vi "NEW数据采集传输系统.vi"() -> ()   [LabVIEW 2016, in "数据传输系统.lvlib"]
uses:
  <vilib>/Averna/Notify Icon/NotifyIcon.llb/BalloonIcon.ctl
  <vilib>/Utility/miscctls.llb/LVPointTypeDef.ctl
  <vilib>/Utility/config.llb/Read Key (String).vi
  <vilib>/Averna/Notify Icon/NotifyIcon.llb/GetSelectedItemEvent.vi
  <vilib>/Averna/Notify Icon/NotifyIcon.llb/SetVisible.vi
  <vilib>/Averna/Notify Icon/NotifyIcon.llb/SetMenuDefaultItem.vi
  <vilib>/Averna/Notify Icon/NotifyIcon.llb/SetTipText.vi
  <vilib>/Utility/config.llb/NI_LVConfig.lvlib
  data/FreeMem.dll
  <vilib>/Averna/Notify Icon/NotifyIcon.llb/NotifyIcon.lvclass
  <vilib>/ptbypt/NI_PtbyPt.lvlib
panel:
  in  "updateconfiguration":T1={"主机"="27.154.58.30", "用户"="update", "密码"="std23506", "远程路径"="数据传输系统\\平台数据传输系统.exe", "下载文件名"="平台数据传输系统.exe", "软件版本"=""}
  out "标题显示":string
  in  "更新":bool
  out "错误输出":errorcluster
  in  "停止输入":bool caption="停止 2"
  in  "系统编码选择框":string(combo)="地表水质量监测"
  in  "数据发送通道":enum16{"TCP", "VISA"}(ring)
  in  "baud rate":u32=9600 caption="波特率"
  in  "VISA resource name":refnum<visa-resource-name> caption="VISA资源名称"
  in  "实时数据发送时间间隔/min":i32=1
  in  "数据组合发送":bool
  in  "日志、参数发送":bool
  in  "2011发送":bool
  in  "判断数据反馈":bool
  in  "数据发送协议":enum16{"2005-212协议", "2017-212协议"}(ring)=enum."2017-212协议"
  in  "重发时间":T2(ring)
  in  "重发日期":T3(ring)
  in  "开机启动":bool
  in  "确定更改起始时间":bool
  in  "更改起始时间":bool
  in  "数据发送起始时间":timestamp format="%<%.3X\n%Y/%m/%d>T"
  in  "每周自动重发":bool=TRUE
  in  "确定":bool
  in  "返回":bool
  in  "PW":string
  in  "MN":string
  in  "PORT":string
  in  "IP":string
  in  "站点设备":string
  in  "站点名称":string
  out "设置超时时间/min":i32=1
  out "状态信息":T4={"1st Error to Convert "=63, "步骤 "=enum."发送数据", "元素"="实时数据", "TCP服务端掉线计数"=0, "TCP掉线时间节点"="2019/05/08 15:24:17"} {"1st Error to Convert" items=["无错误", "参数错误", "内存已满", "超出区域", "文件结束", "文件已打开", "一般文件IO错误", "未找到文件", "文件权限错误", "磁盘已满", "路径副本", "打开过多文件", "未启用", "未找到资源文件", "无法添加资源", "未找到资源", "未找到图像", "图像内存错误", "画笔不存在", "配置错误类型", "配置未找到解析段", "配置解析错误", "配置内存错误", "错误外部代码格式", "错误外部代码偏移量", "外部代码不存在", "空窗口", "销毁窗口错误", "空菜单", "打印已中止", "错误打印记录", "打印驱动程序错误", "打印时窗口错误", "打印时内存错误", "打印对话框错误", "一般打印错误", "无效设备引用句柄", "设备未找到", "设备参数错误", "设备单位错误", "无法打开设备", "设备调用已中止", "一般错误", "用户已取消", "对象ID过低", "对象ID过高", "对象不在堆中", "未知的堆", "错误DefProc ID", "DefProc不在表格中", "范围外信息", "空方法", "未知信息", "不支持管理器调用", "错误地址", "连接过程中", "连接超时", "连接过程中", "不支持网络属性", "网络错误", "正在使用的地址", "系统缺少内存", "连接已中止", "连接已拒绝", "连接未建立", "连接已建立", "连接已关闭", "初始化错误（交互应用程序管理器）", "错误事件发生", "等待无约束事件发生处理程序", "事件发生队列溢出", "错误路径", "未发出信号量", "未识别类型（交互应用程序管理器）"]}
  out "数据接收超时指示灯":bool
  out "空闲时间/s":string
  out "系统时间":string
  out "实时小时数据上传":bool
  out "系统状态改变":bool
  out "软件版本":string
  out "掉线指示":bool
  out "核查数据上传":bool
  out "配置信息":T5
  in  "参数配置":bool
  out "反控数据发送":bool
  out "读取报文显示":string
  out "发送报文显示":string
  out "心跳包":bool
  out "通信状态":bool
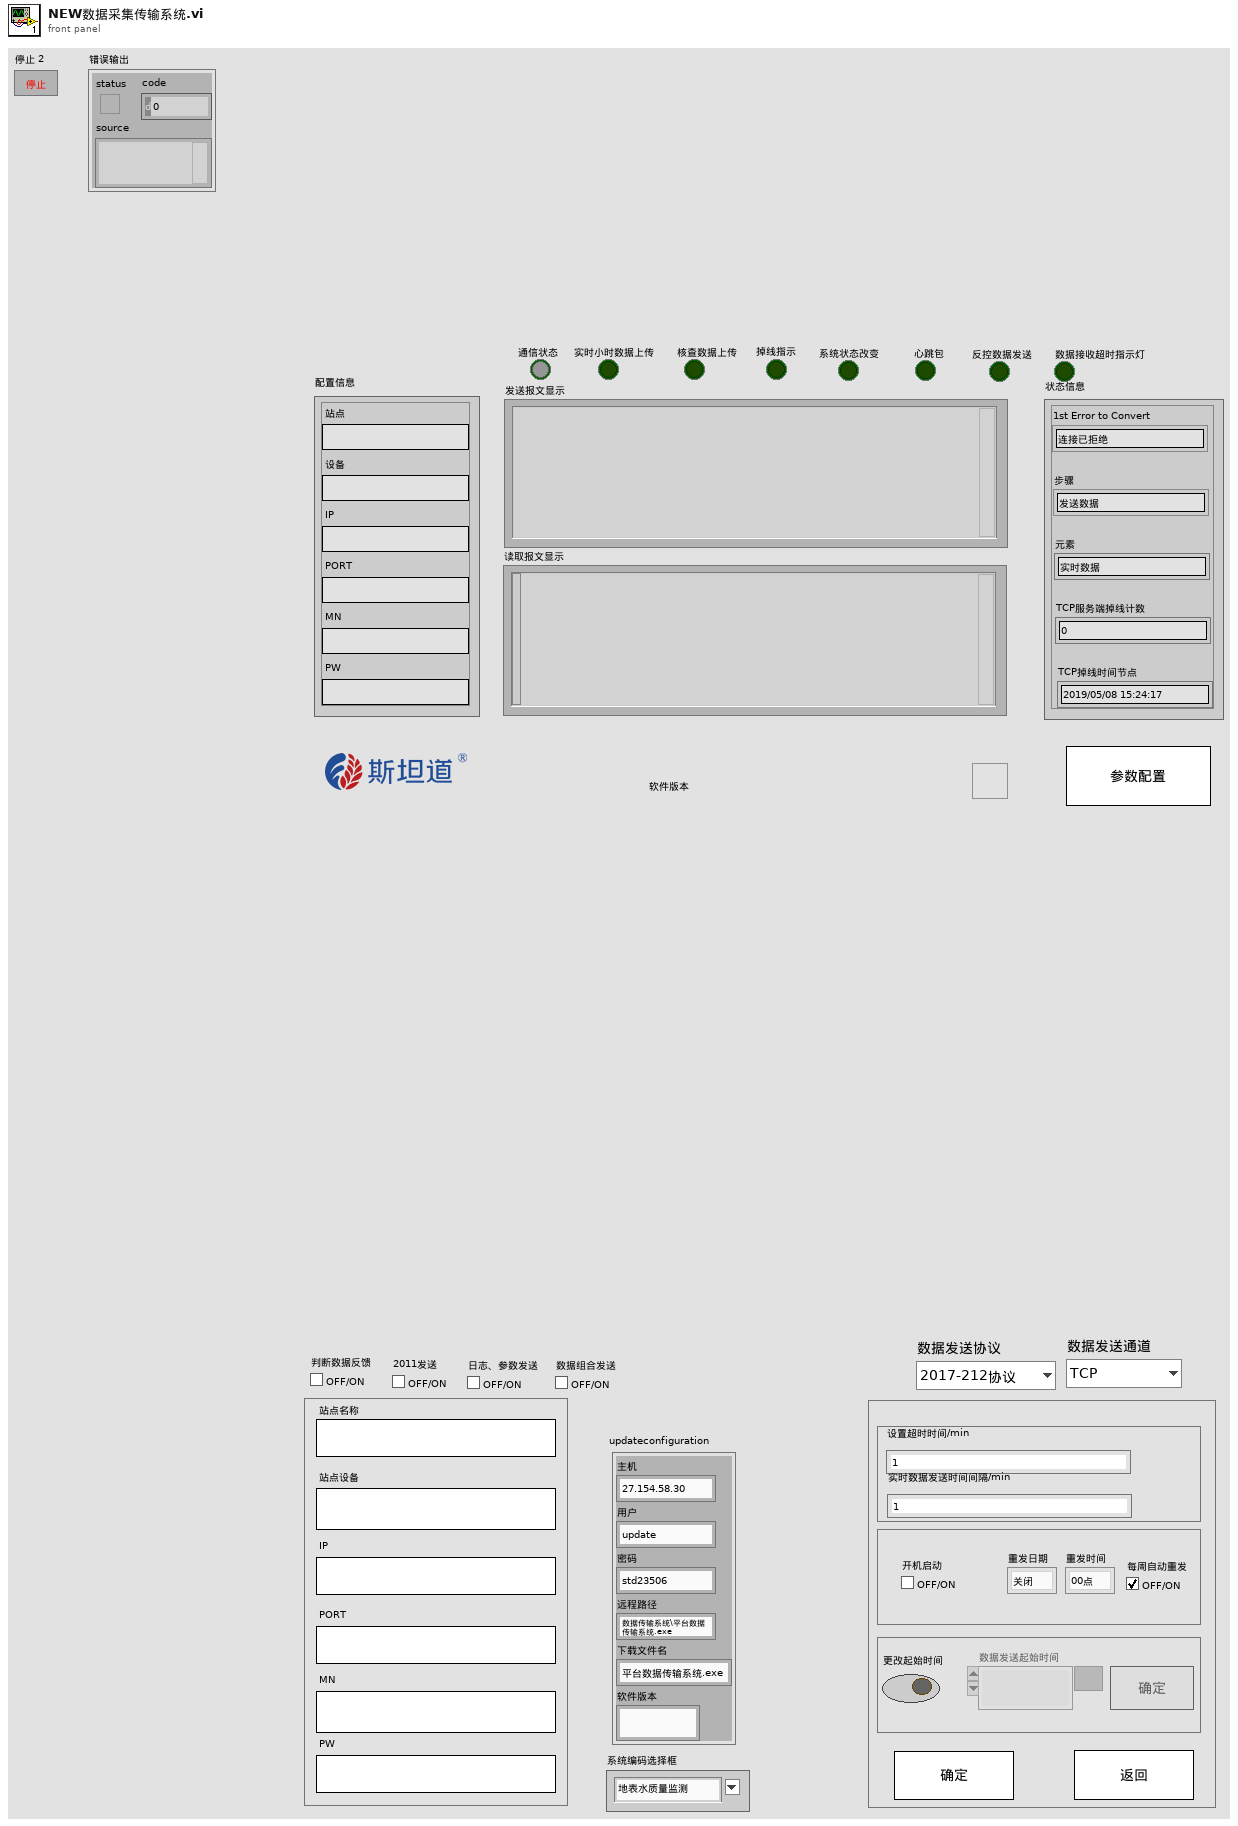
[diagram p1: front panel]
types:
  T1 = cluster{"主机":string, "用户":string, "密码":string, "远程路径":string, "下载文件名":string, "软件版本":string}
  T2 = enum16{"00点", "01点", "02点", "03点", "04点", "05点", "06点", "07点", "08点", "09点", "10点", "11点", "12点", "13点", "14点", "15点", "16点", "17点", "18点", "19点", "20点", "21点", "22点", "23点"}
  T3 = enum16{"关闭", "星期日", "星期一", "星期二", "星期三", "星期四", "星期五", "星期六"}
  T4 = cluster{"1st Error to Convert ":i32, "步骤 ":enum16{"打开连接", "发送数据", "读取数据", "数据处理", "关闭连接"}, "元素":string, "TCP服务端掉线计数":i32, "TCP掉线时间节点":string}
  T5 = cluster{"站点":string, "设备":string, "IP":string, "PORT":string, "MN":string, "PW":string}
  T6 = typedef "LVDateTimeRec.ctl" = cluster{"秒数的小数部分":dbl, "秒":i32, "分":i32, "时":i32, "日":i32, "月":i32, "年":i32, "天数（周）":i32, "天数（年）":i32, "DST":i32}
  T7 = enum32{"invalid app kind", "Development System", "Run Time System", "Student Edition", "Embedded LabVIEW", "Evaluation", "Custom"}
  T8 = typedef "LVPointTypeDef.ctl" = cluster{"Horizontal":i16, "Vertical":i16}
  T9 = cluster{"CODMn":bool, "CODCr":bool, "DO":bool, "铜":bool, "PH":bool, "氨氮":bool, "比电导率":bool, "水温":bool, "COD":bool, "浊度":bool, "总氮":bool, "总磷":bool, "叶绿素a":bool, "藻密度":bool, "水位":bool, "流速":bool, "瞬时流量":bool, "累积流量":bool, "亚硝酸盐":bool, "硫化物":bool, "ORP":bool, "铅":bool, "镉":bool, "锌":bool, "镍":bool, "锰":bool, "汞":bool}
  T10 = typedef "NI_LVConfig.lvlib/Config Data RefNum.ctl" = refnum<k1>
  T11 = typedef "imagedata.ctl" = cluster{"image type":i32, "image depth":i32, "image":u8[], "mask":u8[], "colors":u32[], "Rectangle":cluster{"left":i16, "top":i16, "right":i16, "bottom":i16}}
  T12 = cluster{"[0]":string, "[1]":string, "[2]":string, "[3]":string, "[4]":string, "[5]":string, "[6]":string, "[7]":string, "[8]":string, "[9]":string, "[10]":string, "[11]":string, "[12]":string, "[13]":string, "[14]":string, "[15]":string, "[16]":string, "[17]":string, "[18]":string, "[19]":string, "[20]":string, "[21]":string, "[22]":string, "[23]":string, "[24]":string, "[25]":string, "[26]":string}
  T13 = enum8{"Enabled", "Disabled", "Disabled and Grayed Out"}
  T14 = cluster{"[0]":string, "[1]":string, "[2]":string, "[3]":string, "[4]":string, "[5]":string, "[6]":string, "[7]":string}
  T15 = cluster{"[0]":string, "[1]":string, "[2]":string, "[3]":string, "[4]":string, "[5]":string, "[6]":string, "[7]":string, "[8]":string, "[9]":string, "[10]":string, "[11]":string, "[12]":string, "[13]":string, "[14]":string}
  T16 = enum32{"Invalid", "Standard", "Closed", "Hidden", "Minimized", "Maximized"}
  T17 = typedef "NotifyIcon.lvlib/NotifyIcon.lvclass/BalloonIcon.ctl" = enum32{"None", "Information", "Warning", "Error"}
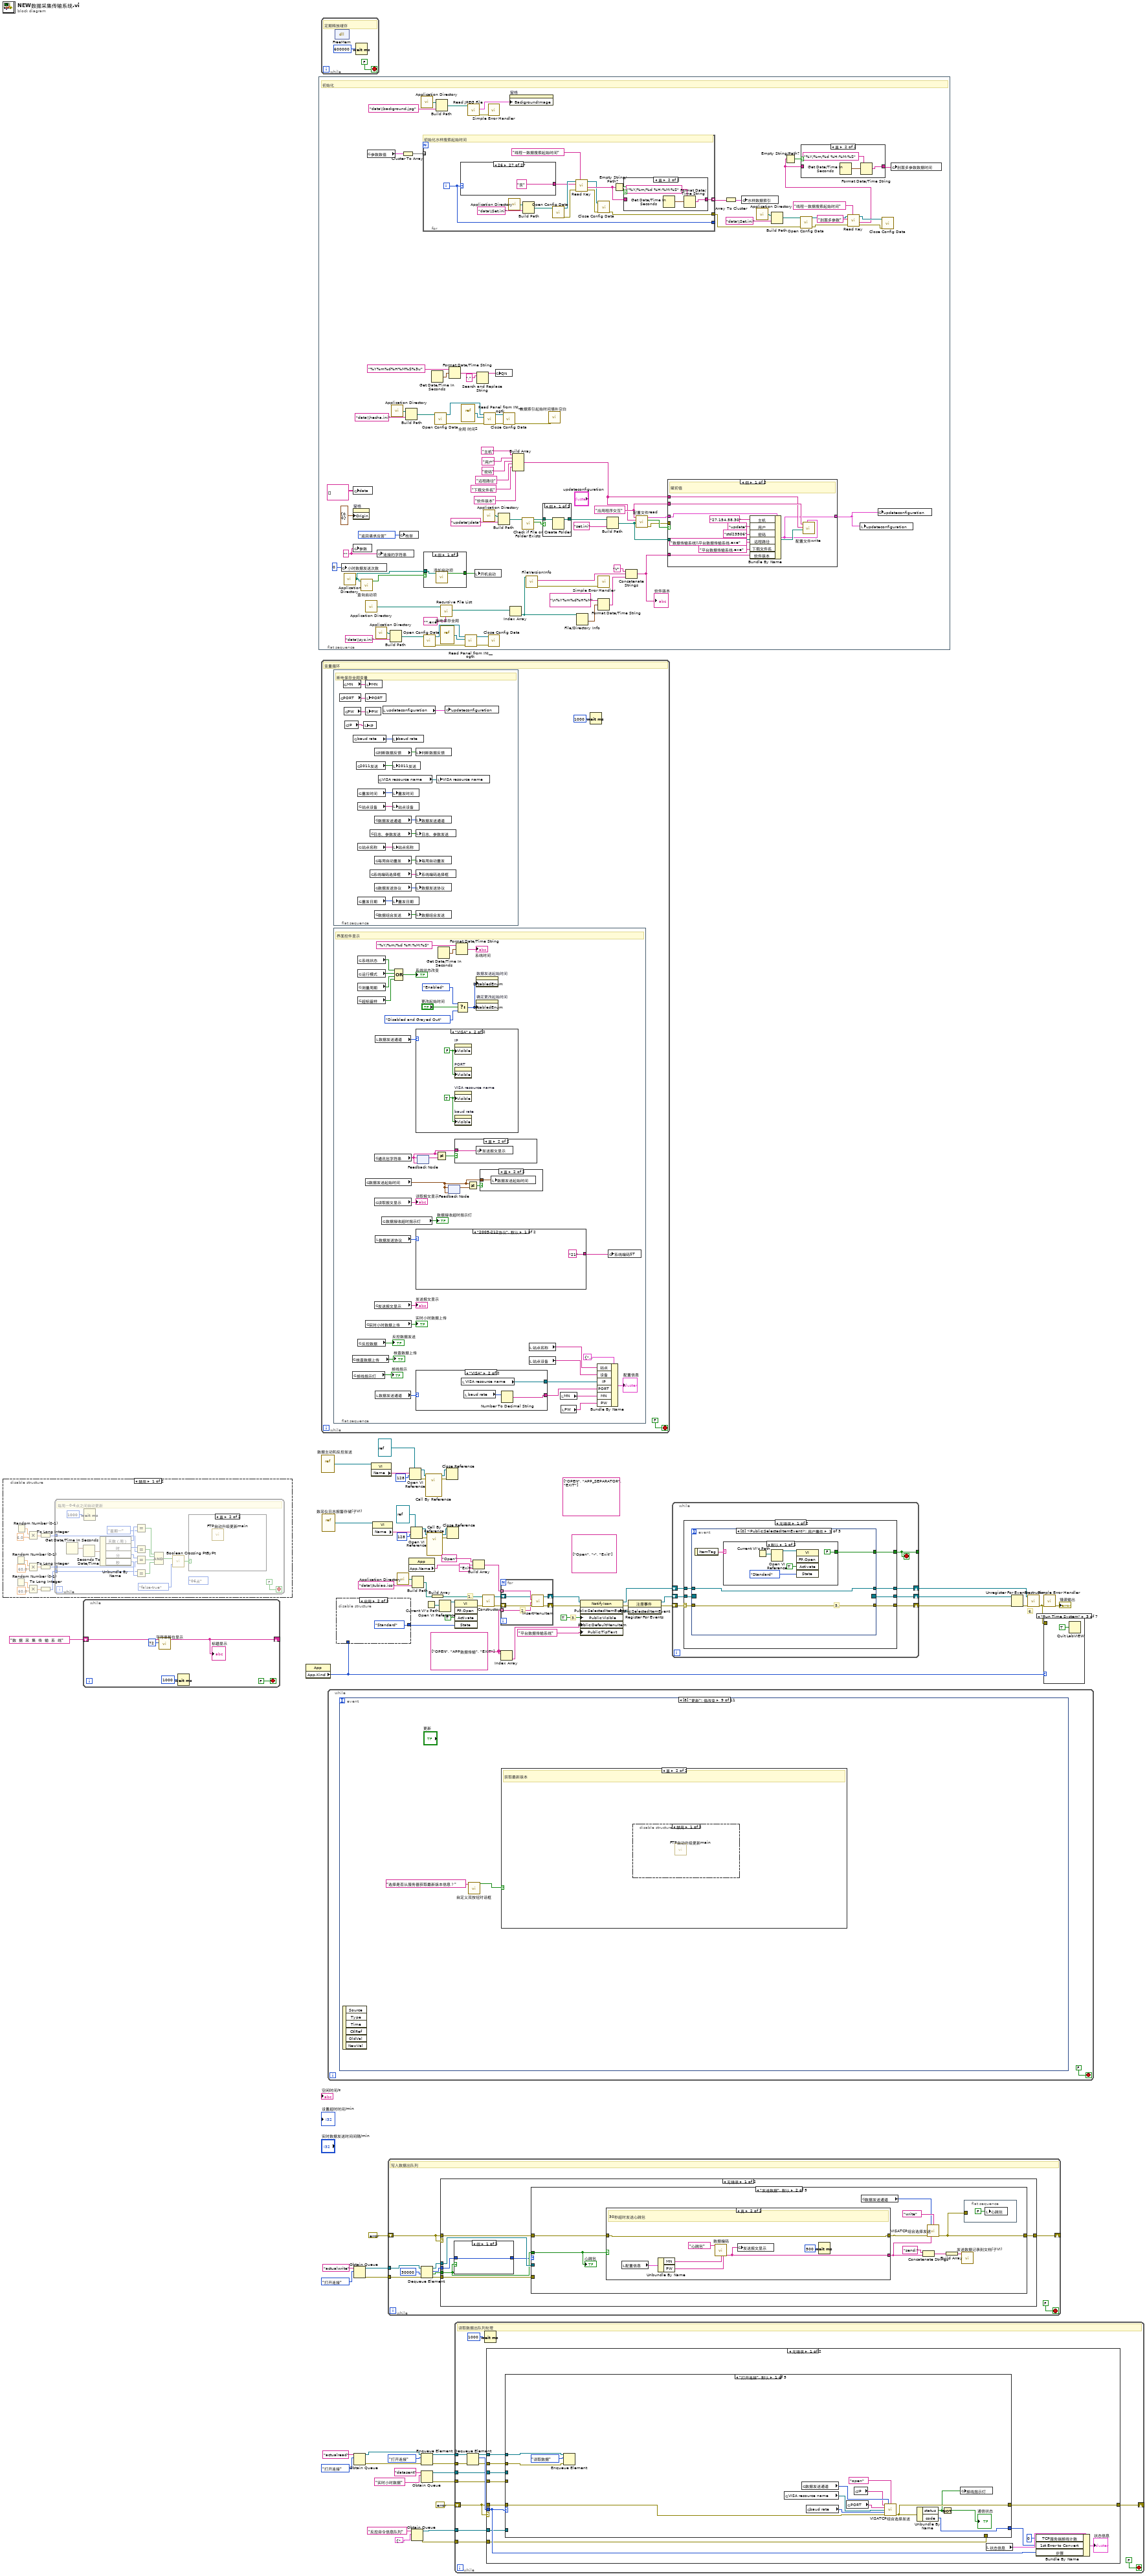
[diagram p0: block diagram]
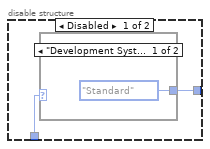
[diagram p4: hidden frame]
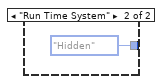
[diagram p5: hidden frame]
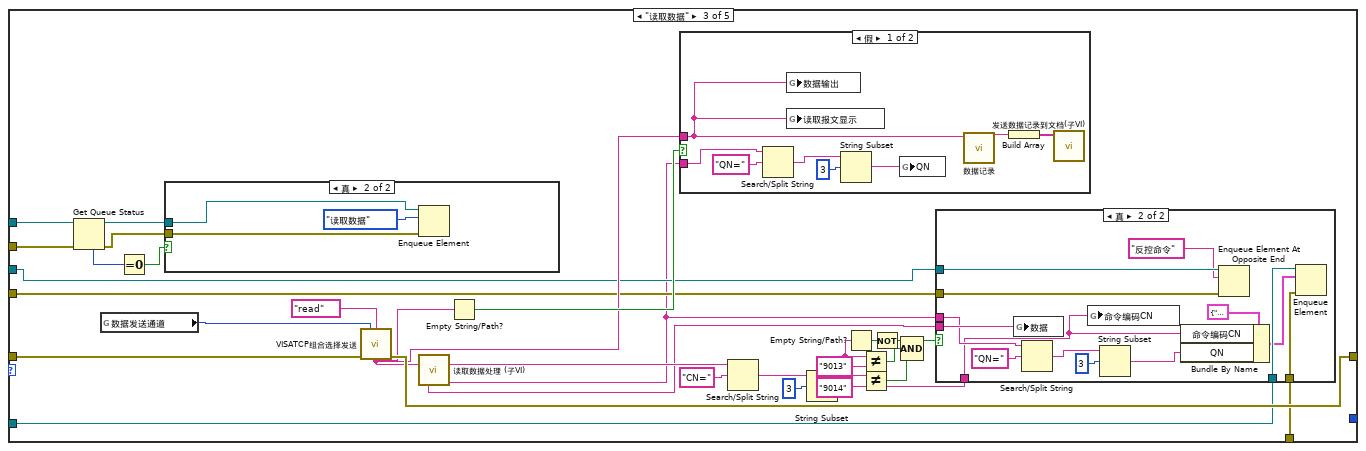
[diagram p7: hidden frame]
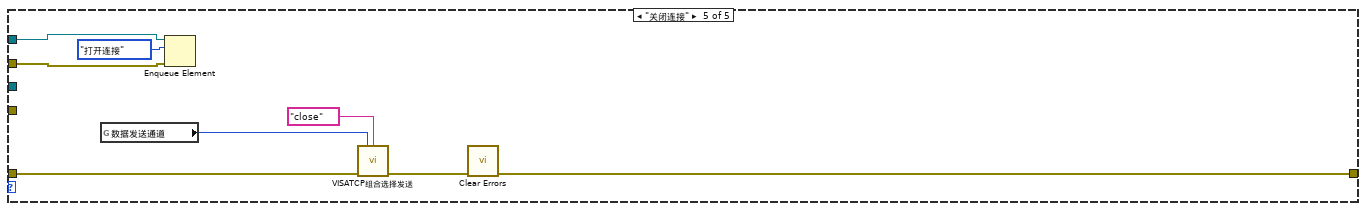
[diagram p12: hidden frame]
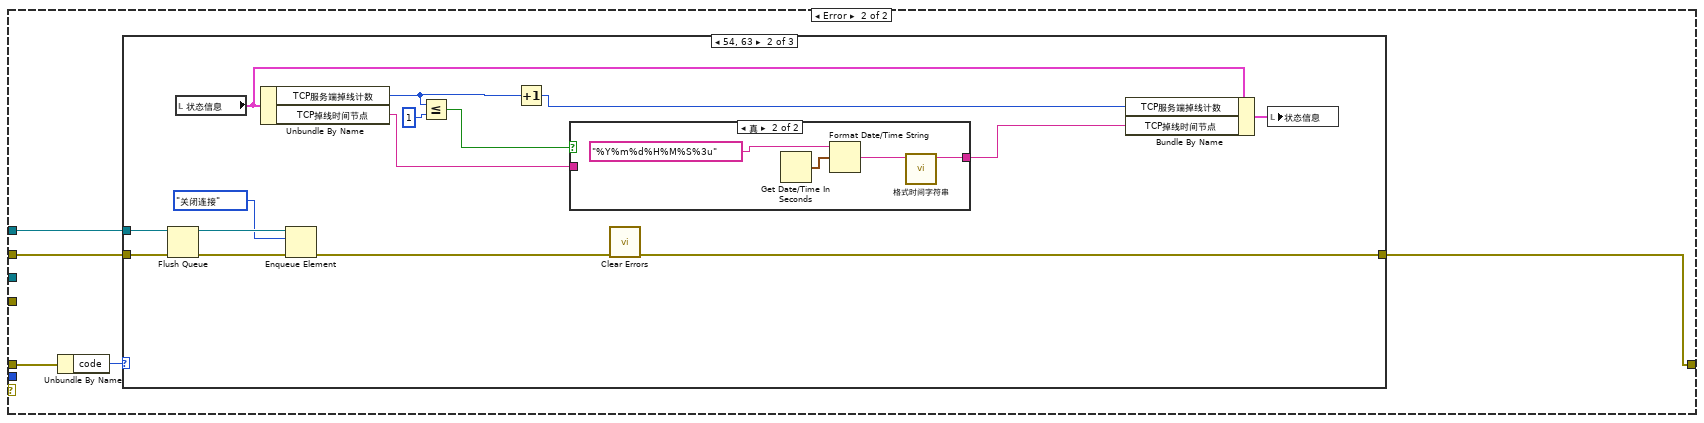
[diagram p13: hidden frame]
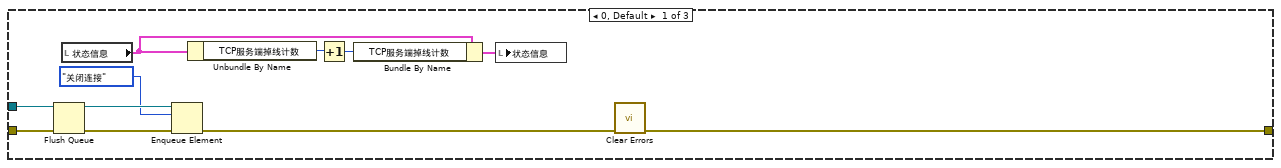
[diagram p14: hidden frame]
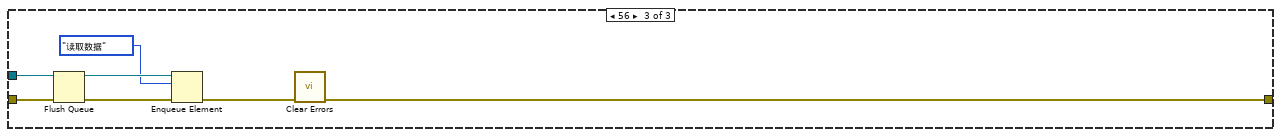
[diagram p16: hidden frame]
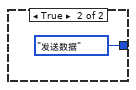
[diagram p17: hidden frame]
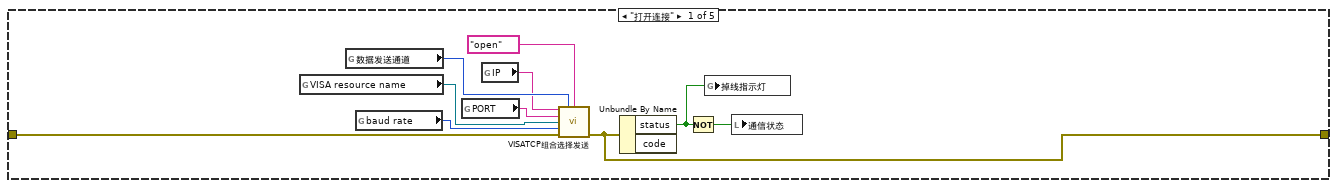
[diagram p18: hidden frame]
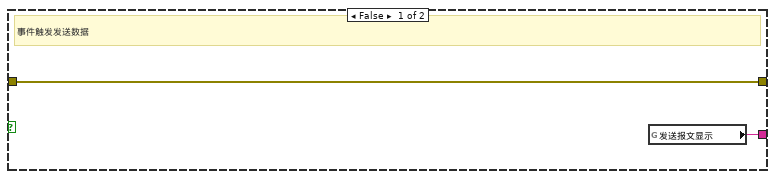
[diagram p19: hidden frame]
diagram:
  w1 = string[] ["OPEN", "APP数据传输", "EXIT"]
  (unwired) string[] ["OPEN", "APP_SEPARATOR", "EXIT"]
  (unwired) string[] ["Open", "-", "Exit"]
  # "6."
  # "3."
  # "1."
  n1 = disable-structure shown="禁用" {
    frame Disabled {
      n2 = Random Number (0-1)() -> (number: 0 to 1=w80:dbl)
      n3 = Random Number (0-1)() -> (number: 0 to 1=w79:dbl)
      n4 = Random Number (0-1)() -> (number: 0 to 1=w83:dbl)
      n5 = Multiply(x=w83, y=6.0) -> (x*y=w77:dbl)
      n6 = Multiply(x=w80, y=60.0) -> (x*y=w75:dbl)
      n7 = Multiply(x=w79, y=60.0) -> (x*y=w73:dbl)
      n8 = To Long Integer(number=w77) -> (32bit integer=w76:i32)
      n9 = To Long Integer(number=w75) -> (32bit integer=w74:i32)
      n10 = To Long Integer(number=w73) -> (32bit integer=w72:i32)
      n11 = while {
        tunnel: w76 -> [w91]
        tunnel: w74 -> [w86]
        tunnel: w72 -> [w85]
        stop <- FALSE stop-if-true
        (unwired) T2."06点" ("重发时间")
        # "每周一0-6点之间自动更新"
        n12 = Get Date/Time In Seconds() -> (seconds since 1Jan1904=w100:timestamp)
        n13 = Seconds To Date/Time(time stamp (now)=w100) -> (date time rec=w96:T6)  [unwired: 1 in]
        n14 = Wait (ms)(milliseconds to wait=u32 1000 ("等待时间（毫秒）")) -> ()  [unwired: 1 out]
        n15 = Unbundle By Name(w96) -> ("天数（周）"=w99:i32, "时"=w93:i32, "分"=w90:i32, "秒"=w88:i32)
        n16 = Equal?(x=w99, y=T3."星期一" ("重发日期")) -> (x = y?=w98:bool)
        n17 = Equal?(x=w93, y=w91) -> (x = y?=w97:bool)
        n18 = Equal?(x=w90, y=w86) -> (x = y?=w89:bool)
        n19 = Equal?(x=w85, y=w88) -> (x = y?=w87:bool)
        n20 = Compound Arithmetic op=AND ("复合运算")(w98, w97, w89, w87) -> (w95:bool)
        n21 = call <vilib>:"Boolean Crossing PtByPt.vi"("direction"=enum16{"either", "false-true", "true-false"}."false-true", "input"=w95) -> ("crossing"=w84:bool)  [unwired: 1 in]
        n22 = case shown="真" w84 {
          frame False {
          }
          frame True {
            n23 = call "FTP自动升级更新main.vi"() -> ()  [unwired: 12 in]
          }
        }
      }
    }
    frame Enabled {
    }
  }
  n24 = while {
    shift-right: [w104] -> _
    shift-left: "数  据  采  集  传  输  系  统" ("标题显示") -> [w105]
    stop <- FALSE stop-if-true
    n25 = call "字符串移位显示.vi"("字符框大小"=72, "字符串输入"=w105) -> ("移位后字符串"=w104:string)  [unwired: 8 in, 1 out]
    "标题显示" <- w104
    n26 = Wait (ms)(milliseconds to wait=u32 1000 ("等待时间（毫秒）")) -> ()  [unwired: 1 out]
  }
  n27 = property class="App"() -> ("App.Kind"=w46:T7)  [unwired: 2 in, 2 out]
  n28 = flat-sequence {
    frame #0 {
      w140 = "应用程序交互" ("section")
      w188 = "" ("参数")
      # "初始化"
      n29 = global write "全局 小时数据发送次数.vi" "小时数据发送次数"(0 ("数值")) -> ()
      n30 = call <vilib>:"Application Directory.vi"() -> ("Application Directory"=w109:path)
      n31 = global write "全局 实时数据参数.vi" "data"(string[][] [] ("data")) -> ()
      n32 = property on="窗格" class="Pane"("Origin"=T8 {"Horizontal"=0, "Vertical"=0} ("原点")) -> ()  [unwired: 2 in, 2 out]
      n33 = global write "全局 实时数据参数.vi" "参数"(w188) -> ()
      n34 = call "查询启动项.vi"("启动文件路径"=w109) -> ("包含启动项"=w110:bool)  [unwired: 9 in, 1 out]
      n35 = call <vilib>:"Application Directory.vi"() -> ("Application Directory"=w168:path)
      n36 = global read "全局1.vi" "参数数值"() -> (w146:T9)
      n37 = call <vilib>:"Application Directory.vi"() -> ("Application Directory"=w162:path)
      n38 = global write "全局 实时数据参数.vi" "连接的字符串"(w188) -> ()
      n39 = Build Path(base path=w162, name or relative path="data\\sys.ini" ("名称或相对路径")) -> (appended path=w160:path)
      n40 = call <vilib>:"Application Directory.vi"() -> ("Application Directory"=w154:path)
      n41 = global write "全局1.vi" "枚举"(enum16{"返回请求应答", "上传数据", "返回执行结果"}."返回请求应答" ("枚举")) -> ()
      n42 = Cluster To Array(cluster=w146) -> (array=w147:bool[])
      n43 = Build Path(base path=w154, name or relative path="data\\hecha.ini" ("名称或相对路径")) -> (appended path=w156:path)
      n44 = call <vilib>:"Application Directory.vi"() -> ("Application Directory"=w179:path)
      n45 = for {
        tunnel: w147 -> [_] mode=indexing
        tunnel: [w223] -> _
        tunnel: [w220] -> w145 mode=indexing
        tunnel: [w219] -> w120
        i -> [w223]
        # "初始化水样搜索起始时间"
        n46 = case shown="26" w223 {
          tunnel: ["CODMn" "CODCr" "DO" "铜" "PH" "氨氮" "比电导率" "水温" "COD" "浊度" "总氮" "总磷" "叶绿素a" "藻密度" "水位" "流速" "瞬时流量" "累积流量" "亚硝氮" "硫化物" "ORP" "铅" "镉" "锌" "镍" "锰" "汞"] -> w226
          frame 0, Default {
          }
          frame 1 {
          }
          frame 2 {
          }
          frame 3 {
          }
          frame 4 {
          }
          frame 5 {
          }
          frame 6 {
          }
          frame 7 {
          }
          frame 8 {
          }
          frame 9 {
          }
          frame 10 {
          }
          frame 11 {
          }
          frame 12 {
          }
          frame 13 {
          }
          frame 14 {
          }
          frame 15 {
          }
          frame 16 {
          }
          frame 17 {
          }
          frame 18 {
          }
          frame 19 {
          }
          frame 20 {
          }
          frame 21 {
          }
          frame 22 {
          }
          frame 23 {
          }
          frame 24 {
          }
          frame 25 {
          }
          frame 26 {
          }
        }
        n47 = call <vilib>:"Application Directory.vi"() -> ("Application Directory"=w232:path)
        n48 = Build Path(base path=w232, name or relative path="data\\Set.ini" ("名称或相对路径")) -> (appended path=w230:path)
        n49 = call <vilib>:"Open Config Data.vi"("configuration file path"=w230) -> ("error out"=w228:errorcluster, "refnum"=w229:T10)  [unwired: 8 in, 1 out]
        n50 = call-poly <vilib>:"Read Key.vi"("section"="线程一数据搜索起始时间", "error in (no error)"=w228, "key"=w226, "refnum"=w229) -> ("error out"=w221:errorcluster, "value"=w224:string, "refnum out"=w222:T10)  [unwired: 4 in, 1 out]
        n51 = call <vilib>:"Close Config Data.vi"("error in (no error)"=w221, "refnum"=w222) -> ("error out"=w219:errorcluster)  [unwired: 8 in, 1 out]
        n52 = Empty String/Path?(string/path=w224) -> (empty?=w225:bool)
        n53 = case shown="真" w225 {
          tunnel: [w233 w234] -> w220
          tunnel: w224 -> [w233 _]
          frame False {
          }
          frame True {
            n54 = Get Date/Time In Seconds() -> (seconds since 1Jan1904=w236:timestamp)
            n55 = Format Date/Time String(time format string (%c)="%Y/%m/%d %H:%M:%S" ("时间格式字符串(%c)"), seconds (now)=w236) -> (date/time string=w234:string)  [unwired: 1 in]
          }
        }
      }
      n56 = call <vilib>:"Open Config Data.vi"("configuration file path"=w160) -> ("error out"=w166:errorcluster, "refnum"=w165:T10)  [unwired: 8 in, 1 out]
      n57 = case shown="假" w110 {
        selector: w110 -> [_ w193]
        tunnel: w109 -> [w192 _]
        tunnel: [w191 w193] -> w108
        frame False {
          n58 = call "添加启动项.vi"("启动文件路径"=w192) -> ("添加成功标记"=w191:bool)  [unwired: 9 in, 1 out]
        }
        frame True {
        }
      }
      n59 = Get Date/Time In Seconds() -> (seconds since 1Jan1904=w184:timestamp)
      n60 = call <vilib>:"Open Config Data.vi"("configuration file path"=w156) -> ("error out"=w150:errorcluster, "refnum"=w151:T10)  [unwired: 8 in, 1 out]
      n61 = Build Path(base path=w179, name or relative path="data\\background.jpg" ("名称或相对路径")) -> (appended path=w178:path)
      n62 = call <vilib>:"Recursive File List.vi"("pattern"="*.exe", "Folder Path"=w168) -> ("All Files in Dir"=w174:path[])  [unwired: 5 in, 4 out]
      n63 = vi-ref "断电保存全局.vi"() -> (w164:refnum<vi>)
      n64 = Format Date/Time String(time format string (%c)="%Y%m%d%H%M%S%3u" ("时间格式字符串(%c)"), seconds (now)=w184) -> (date/time string=w183:string)  [unwired: 1 in]
      n65 = vi-ref "全局 时间2.vi"() -> (w152:refnum<vi>)
      n66 = call <userlib>:"Read Panel from INI__ogtk.vi"("error in (no error)"=w166, "VI ref"=w164, "refnum"=w165) -> ("error out"=w159:errorcluster, "refnum out"=w163:T10)  [unwired: 7 in]
      n67 = call <vilib>:"Read JPEG File.vi"("path to JPEG file"=w178) -> ("error out"=w176:errorcluster, "image data"=w177:T11)  [unwired: 8 in, 1 out]
      n68 = local write "开机启动"(w108) -> ()
      n69 = Search and Replace String(input string=w183, search string="." ("搜索字符串")) -> (result string=w181:string)  [unwired: 6 in, 3 out]
      n70 = call <vilib>:"Application Directory.vi"() -> ("Application Directory"=w126:path)
      n71 = call <userlib>:"Read Panel from INI__ogtk.vi"("error in (no error)"=w150, "VI ref"=w152, "refnum"=w151) -> ("error out"=w149:errorcluster, "refnum out"=w153:T10)  [unwired: 7 in]
      n72 = call <vilib>:"Simple Error Handler.vi"("error in (no error)"=w176) -> ()  [unwired: 4 in, 5 out]
      n73 = call <vilib>:"Close Config Data.vi"("error in (no error)"=w159, "refnum"=w163) -> ()  [unwired: 8 in, 2 out]
      n74 = global write "全局1.vi" "QN"(w181) -> ()
      n75 = Build Path(base path=w126, name or relative path="update\\data" ("名称或相对路径")) -> (appended path=w127:path)
      n76 = call <vilib>:"Close Config Data.vi"("error in (no error)"=w149, "refnum"=w153) -> ("error out"=w148:errorcluster)  [unwired: 8 in, 1 out]
      n77 = property on="窗格" class="Pane"("BackgroundImage"=w177) -> ()  [unwired: 2 in, 2 out]
      n78 = Index Array(array=w174) -> (element=w173:path)  [unwired: 1 in]
      n79 = Build Array("主机" ("section"), "用户" ("section"), "密码" ("key"), "远程路径" ("key"), "下载文件名" ("key"), "软件版本" ("key")) -> (w130:string[])
      n80 = call <vilib>:"Check if File or Folder Exists.vi"("path"=w127) -> ("file or folder exists?"=w128:bool, "dup path"=w129:path)  [unwired: 8 in, 1 out]
      n81 = call <vilib>:"FileVersionInfo.vi"("Application Path in"=w173) -> ("error out"=w167:errorcluster, "File Version Info"=w157:string)  [unwired: 7 in, 2 out]
      n82 = case shown="假" w128 {
        tunnel: w129 -> [w199 w200]
        tunnel: [w198 w200] -> w124
        frame False {
          n83 = Create Folder(path (use dialog)=w199) -> (created path=w198:path)  [unwired: 2 in, 2 out]
        }
        frame True {
        }
      }
      n84 = call "数据索引起始时间填补空白.vi"("error in (no error)"=w148) -> ()  [unwired: 10 in, 1 out]
      n85 = File/Directory Info(path=w173) -> (last mod=w172:timestamp)  [unwired: 1 in, 6 out]
      n86 = call <vilib>:"Simple Error Handler.vi"("error in (no error)"=w167) -> ()  [unwired: 4 in, 5 out]
      n87 = Format Date/Time String(time format string (%c)="\n%Y%m%d%H%M" ("时间格式字符串(%c)"), seconds (now)=w172) -> (date/time string=w169:string)  [unwired: 1 in]
      n88 = Build Path(base path=w124, name or relative path="set.ini" ("名称或相对路径")) -> (appended path=w139:path)
      n89 = Concatenate Strings("V" ("字符串"), w157, w169) -> (w141:string)
      "软件版本" <- w141
      n90 = call "配置文件read.vi"("configuration file path"=w139, "键数组"=w130, "段"=w140) -> ("error out"=w138:errorcluster, "section exists?"=w143:bool, "updateconfiguration"=w142:T1)  [unwired: 6 in]
      n91 = case shown="假" w143 {
        tunnel: w142 -> [w207 w213]
        tunnel: [w206 w212] -> w137
        tunnel: w141 -> [w201 w218]
        tunnel: w140 -> [w210 w217]
        tunnel: w130 -> [w209 w216]
        tunnel: w139 -> [w208 w215]
        tunnel: w138 -> [_ w214]
        frame False {
          # "赋初值"
          n92 = Bundle By Name(cluster=w207, "主机"="27.154.58.30" ("key"), "用户"="update", "密码"="std23506", "远程路径"="数据传输系统\\平台数据传输系统.exe", "下载文件名"="平台数据传输系统.exe", "软件版本"=w201) -> (w206:T1)
          n93 = call "配置文件write.vi"("updateconfiguration"=w206, "configuration file path"=w208, "键数组"=w209, "段"=w210) -> ()  [unwired: 7 in, 1 out]
        }
        frame True {
          # "本地"
          n94 = Bundle By Name(cluster=w213, "软件版本"=w218) -> (w212:T1)
          n95 = call "配置文件write.vi"("updateconfiguration"=w212, "error in (no error)"=w214, "configuration file path"=w215, "键数组"=w216, "段"=w217) -> ()  [unwired: 6 in, 1 out]
        }
      }
      n96 = Array To Cluster(array=w145) -> (cluster=w144:T12)
      n97 = global write "全局 水样时间.vi" "水样数据索引"(w144) -> ()
      n98 = call <vilib>:"Application Directory.vi"() -> ("Application Directory"=w123:path)
      n99 = Build Path(base path=w123, name or relative path="data\\Set.ini" ("名称或相对路径")) -> (appended path=w121:path)
      n100 = call <vilib>:"Open Config Data.vi"("error in (no error)"=w120, "configuration file path"=w121) -> ("error out"=w117:errorcluster, "refnum"=w118:T10)  [unwired: 7 in, 1 out]
      n101 = call-poly <vilib>:"Read Key.vi"("section"="线程一数据搜索起始时间", "error in (no error)"=w117, "key"="剖面多参数", "refnum"=w118) -> ("error out"=w114:errorcluster, "value"=w112:string, "refnum out"=w115:T10)  [unwired: 4 in, 1 out]
      n102 = Empty String/Path?(string/path=w112) -> (empty?=w111:bool)
      n103 = case shown="真" w111 {
        tunnel: [w194 w195] -> w113
        tunnel: w112 -> [w194 _]
        frame False {
        }
        frame True {
          n104 = Get Date/Time In Seconds() -> (seconds since 1Jan1904=w197:timestamp)
          n105 = Format Date/Time String(time format string (%c)="%Y/%m/%d %H:%M:%S" ("时间格式字符串(%c)"), seconds (now)=w197) -> (date/time string=w195:string)  [unwired: 1 in]
        }
      }
      n106 = local write "updateconfiguration"(w137) -> ()
      n107 = global write "update全局.vi" "updateconfiguration"(w137) -> ()
      n108 = call <vilib>:"Close Config Data.vi"("error in (no error)"=w114, "refnum"=w115) -> ()  [unwired: 8 in, 2 out]
      n109 = global write "全局 水样时间.vi" "剖面多参数数据时间"(w113) -> ()
    }
  }
  n110 = while {
    stop <- FALSE stop-if-true
    # "定期释放缓存"
    n111 = dll-call lib="PTH2habs F\tgitkrakenCC=平台数采程序 - V2.0.1-芜湖污染源数据传输标准dataFreeMem.dll" fn="FreeMem"() -> ()  [unwired: 4 in, 2 out]
    n112 = Wait (ms)(milliseconds to wait=u32 600000 ("等待时间（毫秒）")) -> ()  [unwired: 1 out]
  }
  n113 = while {
    stop <- FALSE stop-if-true
    # "变量循环"
    n114 = flat-sequence {
      frame #0 {
        # "断电保存全局变量"
        n115 = global read "断电保存全局.vi" "PORT"() -> (w337:string)
        n116 = global read "断电保存全局.vi" "MN"() -> (w336:string)
        n117 = global read "断电保存全局.vi" "PW"() -> (w335:string)
        n118 = global read "断电保存全局.vi" "IP"() -> (w338:string)
        n119 = global read "断电保存全局.vi" "baud rate"() -> (w333:u32)
        n120 = global read "断电保存全局.vi" "2011发送"() -> (w329:bool)
        n121 = global read "断电保存全局.vi" "重发时间"() -> (w323:T2)
        n122 = global read "断电保存全局.vi" "站点设备"() -> (w339:string)
        n123 = global read "断电保存全局.vi" "站点名称"() -> (w340:string)
        n124 = global read "断电保存全局.vi" "重发日期"() -> (w331:T3)
        n125 = local write "IP"(w338) -> ()
        n126 = local write "MN"(w336) -> ()
        n127 = local write "PORT"(w337) -> ()
        n128 = local write "PW"(w335) -> ()
        n129 = global read "断电保存全局.vi" "日志、参数发送"() -> (w328:bool)
        n130 = global read "断电保存全局.vi" "系统编码选择框"() -> (w324:string)
        n131 = global read "断电保存全局.vi" "判断数据反馈"() -> (w330:bool)
        n132 = global read "断电保存全局.vi" "数据发送通道"() -> (w325:enum16{"TCP", "VISA"})
        n133 = global read "断电保存全局.vi" "每周自动重发"() -> (w332:bool)
        n134 = global read "断电保存全局.vi" "数据发送协议"() -> (w326:enum16{"2005-212协议", "2017-212协议"})
        n135 = global read "断电保存全局.vi" "数据组合发送"() -> (w327:bool)
        n136 = global read "断电保存全局.vi" "VISA resource name"() -> (w334:refnum<visa-resource-name>)
        n137 = local read "updateconfiguration"() -> (w322:T1)
        n138 = local write "baud rate"(w333) -> ()
        n139 = local write "2011发送"(w329) -> ()
        n140 = local write "重发时间"(w323) -> ()
        n141 = local write "站点设备"(w339) -> ()
        n142 = local write "站点名称"(w340) -> ()
        n143 = local write "重发日期"(w331) -> ()
        n144 = local write "判断数据反馈"(w330) -> ()
        n145 = local write "数据发送通道"(w325) -> ()
        n146 = local write "日志、参数发送"(w328) -> ()
        n147 = local write "每周自动重发"(w332) -> ()
        n148 = local write "系统编码选择框"(w324) -> ()
        n149 = local write "数据发送协议"(w326) -> ()
        n150 = local write "数据组合发送"(w327) -> ()
        n151 = local write "VISA resource name"(w334) -> ()
        n152 = global write "update全局.vi" "updateconfiguration"(w322) -> ()
      }
    }
    n153 = flat-sequence {
      frame #0 {
        # "界面控件显示"
        n154 = global read "全局1.vi" "核查数据上传"() -> (→"核查数据上传":bool)
        n155 = global read "全局 数据发送重叠.vi" "掉线指示灯"() -> (→"掉线指示":bool)
        n156 = global read "全局1.vi" "系统状态"() -> (w271:bool)
        n157 = global read "全局1.vi" "运行模式"() -> (w272:bool)
        n158 = global read "全局1.vi" "测量周期"() -> (w273:bool)
        n159 = global read "全局1.vi" "超标留样"() -> (w274:bool)
        n160 = global read "全局1.vi" "反控数据"() -> (→"反控数据发送":bool)
        n161 = global read "全局1.vi" "数据发送起始时间"() -> (w268:timestamp)
        n162 = global read "全局1.vi" "实时小时数据上传"() -> (→"实时小时数据上传":bool)
        n163 = global read "全局1.vi" "通讯包字符串"() -> (w285:string)
        n164 = global read "全局1.vi" "读取报文显示"() -> (→"读取报文显示":string)
        n165 = global read "全局1.vi" "发送报文显示"() -> (→"发送报文显示":string)
        n166 = local read "数据发送通道"() -> (w279:enum16{"TCP", "VISA"})
        n167 = local read "数据发送协议"() -> (w293:enum16{"2005-212协议", "2017-212协议"})
        n168 = local read "数据发送通道"() -> (w304:enum16{"TCP", "VISA"})
        n169 = global read "全局 数据发送重叠.vi" "数据接收超时指示灯"() -> (→"数据接收超时指示灯":bool)
        n170 = Compound Arithmetic op=OR ("复合运算")(w271, w272, w273, w274) -> (→"系统状态改变":bool)
        n171 = case shown="\"VISA\"" w279 {
          frame "TCP", Default {
            w306 = TRUE ("可见")
            w307 = FALSE ("可见")
            n172 = property on="IP" class="Str"("Visible"=w306) -> ()  [unwired: 2 in, 2 out]
            n173 = property on="PORT" class="Str"("Visible"=w306) -> ()  [unwired: 2 in, 2 out]
            n174 = property on="VISA resource name" class="VISAName"("Visible"=w307) -> ()  [unwired: 2 in, 2 out]
            n175 = property on="baud rate" class="DigNum (严格)"("Visible"=w307) -> ()  [unwired: 2 in, 2 out]
          }
          frame "VISA" {
            w308 = FALSE ("可见")
            w309 = TRUE ("可见")
            n176 = property on="IP" class="Str"("Visible"=w308) -> ()  [unwired: 2 in, 2 out]
            n177 = property on="PORT" class="Str"("Visible"=w308) -> ()  [unwired: 2 in, 2 out]
            n178 = property on="VISA resource name" class="VISAName"("Visible"=w309) -> ()  [unwired: 2 in, 2 out]
            n179 = property on="baud rate" class="DigNum (严格)"("Visible"=w309) -> ()  [unwired: 2 in, 2 out]
          }
        }
        n180 = case shown="\"2005-212协议\", 默认" w293 {
          tunnel: ["21" ("设备编码MN") w312] -> w292
          frame "2005-212协议", Default {
          }
          frame "2017-212协议" {
            n181 = global read "断电保存全局.vi" "系统编码选择框"() -> (w313:string)
            n182 = case shown="\"地表水质量监测\", 默认" w313 {
              tunnel: ["52" ("设备编码MN") "32" ("设备编码MN") "21" ("设备编码MN")] -> w312
              frame "污水排放过程监测" {
              }
              frame "地表水体污染源" {
              }
              frame "地表水质量监测", Default {
              }
            }
          }
        }
        n183 = case shown="\"VISA\"" w304 {
          tunnel: [w318 w321] -> w301
          tunnel: [w317 w319] -> w298
          frame "TCP", Default {
            n184 = local read "PORT"() -> (w317:string)
            n185 = local read "IP"() -> (w318:string)
          }
          frame "VISA" {
            n186 = local read "VISA resource name"() -> (w321:refnum<visa-resource-name>)
            n187 = local read "baud rate"() -> (w320:u32)
            n188 = Number To Decimal String(number=w320) -> (decimal integer string=w319:string)  [unwired: 1 in]
          }
        }
        n189 = feedback #1(w285) -> (w286:string)
        n190 = feedback-in #1(w285) -> ()
        n191 = Not Equal?(x=w285, y=w286) -> (x != y?=w284:bool)
        n192 = Get Date/Time In Seconds() -> (seconds since 1Jan1904=w294:timestamp)
        n193 = feedback #2(w268) -> (w270:timestamp)
        n194 = feedback-in #2(w268) -> ()
        n195 = case shown="真" w284 {
          tunnel: w285 -> [_ w310]
          frame False {
          }
          frame True {
            n196 = global write "全局1.vi" "发送报文显示"(w310) -> ()
          }
        }
        n197 = Format Date/Time String(time format string (%c)="%Y/%m/%d %H:%M:%S" ("时间格式字符串(%c)"), seconds (now)=w294) -> (date/time string=→"系统时间":string)  [unwired: 1 in]
        n198 = Select(t=T13."Enabled" ("禁用"), s="更改起始时间", f=T13."Disabled and Grayed Out" ("禁用")) -> (s? t:f=w280:T13)
        n199 = Not Equal?(x=w268, y=w270) -> (x != y?=w269:bool)
        n200 = property on="数据发送起始时间" class="AbsTime (严格)"("DisabledEnum"=w280) -> ()  [unwired: 2 in, 2 out]
        n201 = property on="确定更改起始时间" class="Bool"("DisabledEnum"=w280) -> ()  [unwired: 2 in, 2 out]
        n202 = case shown="真" w269 {
          tunnel: w268 -> [_ w305]
          frame False {
          }
          frame True {
            n203 = local write "数据发送起始时间"(w305) -> ()
          }
        }
        n204 = local read "站点名称"() -> (w300:string)
        n205 = local read "站点设备"() -> (w299:string)
        n206 = local read "MN"() -> (w297:string)
        n207 = local read "PW"() -> (w296:string)
        n208 = Bundle By Name(cluster=T5 {"站点"="", "设备"="", "IP"="", "PORT"="", "MN"="", "PW"=""} ("配置信息"), "站点"=w300, "设备"=w299, "IP"=w301, "PORT"=w298, "MN"=w297, "PW"=w296) -> (→"配置信息":T5)
        n209 = global write "全局1.vi" "系统编码ST"(w292) -> ()
      }
    }
    n210 = Wait (ms)(milliseconds to wait=u32 1000 ("等待时间（毫秒）")) -> ()  [unwired: 1 out]
  }
  n211 = vi-ref "数据主动和反控发送.vi"() -> (w37:refnum<vi>)
  n212 = vi-ref "数采仪日志报警存储(子VI).vi"() -> (w38:refnum<vi>)
  n213 = while {
    stop <- FALSE stop-if-true
    n214 = event shown="[8] \"更新\": 值改变" {
      selector: _ -> [_ _ _ _ _ _ _ _ _ _ _]
      dyn-events: _ -> [_ _ _ _ _ _ _ _ _ _ _]
      timeout: _ -> [_ _ _ _ _ _ _ _ _ _ _]
      event Timeout {
        n215 = event-data() -> ()  [unwired: 1 in, 3 out]
      }
      event "站点名称", "站点设备", "IP", "PORT", "MN", "PW", "VISA resource name", "baud rate", "系统编码选择框", "每周自动重发", "重发日期", "重发时间": Value Change {
        n216 = event-data() -> ()  [unwired: 1 in, 6 out]
        n217 = flat-sequence {
          frame #0 {
            n218 = global write "断电保存全局.vi" "PW"("PW") -> ()
            n219 = global write "断电保存全局.vi" "站点名称"("站点名称") -> ()
            n220 = global write "断电保存全局.vi" "MN"("MN") -> ()
            n221 = global write "断电保存全局.vi" "PORT"("PORT") -> ()
            n222 = global write "断电保存全局.vi" "IP"("IP") -> ()
            n223 = global write "断电保存全局.vi" "重发日期"("重发日期") -> ()
            n224 = global write "断电保存全局.vi" "重发时间"("重发时间") -> ()
            n225 = global write "断电保存全局.vi" "站点设备"("站点设备") -> ()
            n226 = global write "断电保存全局.vi" "baud rate"("baud rate") -> ()
            n227 = global write "断电保存全局.vi" "系统编码选择框"("系统编码选择框") -> ()
            n228 = global write "断电保存全局.vi" "每周自动重发"("每周自动重发") -> ()
            n229 = global write "断电保存全局.vi" "VISA resource name"("VISA resource name") -> ()
          }
          frame #1 {
            n230 = call <vilib>:"Application Directory.vi"() -> ("Application Directory"=w354:path)
            n231 = Build Path(base path=w354, name or relative path="data\\sys.ini" ("名称或相对路径")) -> (appended path=w356:path)
            n232 = call <vilib>:"Open Config Data.vi"("configuration file path"=w356) -> ("error out"=w360:errorcluster, "refnum"=w357:T10)  [unwired: 8 in, 1 out]
            n233 = vi-ref "断电保存全局.vi"() -> (w358:refnum<vi>)
            n234 = call <userlib>:"Write Panel to INI__ogtk.vi"("error in (no error)"=w360, "VI ref"=w358, "refnum"=w357) -> ("error out"=w361:errorcluster, "refnum out"=w359:T10)  [unwired: 7 in]
            n235 = call <vilib>:"Close Config Data.vi"("error in (no error)"=w361, "refnum"=w359) -> ("error out"=w366:errorcluster, "file path"=w367:path)  [unwired: 8 in]
            n236 = Open/Create/Replace File(file path (use dialog)=w367, error in=w366) -> (refnum out=w363:refnum<file>, error out=w362:errorcluster)  [unwired: 4 in, 1 out]
            n237 = Flush File(refnum=w363, error in=w362) -> (refnum out=w364:refnum<file>, error out=w365:errorcluster)
            n238 = Close File(refnum=w364, error in=w365) -> ()  [unwired: 2 out]
          }
        }
      }
      event "数据发送通道", "数据发送协议", "数据组合发送", "2011发送", "日志、参数发送", "判断数据反馈": Value Change {
        n239 = event-data() -> ("CtlRef"=w371:refnum<vi>, "OldVal"=w369:variant, "NewVal"=w368:variant)  [unwired: 1 in, 3 out]
        n240 = property class="Ctl"(reference=w371) -> ("Label.Text"=w370:string)  [unwired: 1 in, 2 out]
        n241 = case shown="\"数据发送通道\"" w370 {
          tunnel: w369 -> [_ w375 w398 w421 w444 w467 w490]
          tunnel: w368 -> [_ w372 w395 w418 w441 w464 w487]
          frame "假", Default {
          }
          frame "数据发送通道" {
            n242 = Variant To Data(type=enum16{"TCP", "VISA"}."TCP" ("数据发送通道"), Variant=w372) -> (data=w373:enum16{"TCP", "VISA"})  [unwired: 1 in, 1 out]
            n243 = global write "断电保存全局.vi" "数据发送通道"(w373) -> ()
            n244 = Two Button Dialog(message="TCP通过网络发送数据，VISA通过串口发送数据，确定更改数据发送通道吗？" ("消息")) -> (T button?=w376:bool)  [unwired: 2 in]
            n245 = case shown="假" w376 {
              tunnel: w375 -> [w379 _]
              frame False {
                n246 = Variant To Data(type=enum16{"TCP", "VISA"}."TCP" ("数据发送通道"), Variant=w379) -> (data=w378:enum16{"TCP", "VISA"})  [unwired: 1 in, 1 out]
                n247 = global write "断电保存全局.vi" "数据发送通道"(w378) -> ()
              }
              frame True {
                n248 = flat-sequence {
                  frame #0 {
                  }
                  frame #1 {
                    n249 = call <vilib>:"Application Directory.vi"() -> ("Application Directory"=w381:path)
                    n250 = Build Path(base path=w381, name or relative path="data\\sys.ini" ("名称或相对路径")) -> (appended path=w383:path)
                    n251 = call <vilib>:"Open Config Data.vi"("configuration file path"=w383) -> ("error out"=w387:errorcluster, "refnum"=w384:T10)  [unwired: 8 in, 1 out]
                    n252 = vi-ref "断电保存全局.vi"() -> (w385:refnum<vi>)
                    n253 = call <userlib>:"Write Panel to INI__ogtk.vi"("error in (no error)"=w387, "VI ref"=w385, "refnum"=w384) -> ("error out"=w388:errorcluster, "refnum out"=w386:T10)  [unwired: 7 in]
                    n254 = call <vilib>:"Close Config Data.vi"("error in (no error)"=w388, "refnum"=w386) -> ("error out"=w393:errorcluster, "file path"=w394:path)  [unwired: 8 in]
                    n255 = Open/Create/Replace File(file path (use dialog)=w394, error in=w393) -> (refnum out=w390:refnum<file>, error out=w389:errorcluster)  [unwired: 4 in, 1 out]
                    n256 = Flush File(refnum=w390, error in=w389) -> (refnum out=w391:refnum<file>, error out=w392:errorcluster)
                    n257 = Close File(refnum=w391, error in=w392) -> ()  [unwired: 2 out]
                  }
                }
              }
            }
          }
          frame "数据发送协议" {
            n258 = Variant To Data(type=enum16{"2005-212协议", "2017-212协议"}."2017-212协议" ("数据"), Variant=w395) -> (data=w396:enum16{"2005-212协议", "2017-212协议"})  [unwired: 1 in, 1 out]
            n259 = global write "断电保存全局.vi" "数据发送协议"(w396) -> ()
            n260 = Two Button Dialog(message="2005对应旧版通信协议，2017对应最新版协议，对应协议因子编码会不同，\n更改可能导致数据不能被平台识别，确定更改数据发送协议吗？" ("消息")) -> (T button?=w399:bool)  [unwired: 2 in]
            n261 = case shown="真" w399 {
              tunnel: w398 -> [w403 _]
              frame False {
                n262 = Variant To Data(type=enum16{"2005-212协议", "2017-212协议"}."2017-212协议" ("数据"), Variant=w403) -> (data=w401:enum16{"2005-212协议", "2017-212协议"})  [unwired: 1 in, 1 out]
                n263 = global write "断电保存全局.vi" "数据发送协议"(w401) -> ()
              }
              frame True {
                n264 = flat-sequence {
                  frame #0 {
                  }
                  frame #1 {
                    n265 = call <vilib>:"Application Directory.vi"() -> ("Application Directory"=w404:path)
                    n266 = Build Path(base path=w404, name or relative path="data\\sys.ini" ("名称或相对路径")) -> (appended path=w406:path)
                    n267 = call <vilib>:"Open Config Data.vi"("configuration file path"=w406) -> ("error out"=w410:errorcluster, "refnum"=w407:T10)  [unwired: 8 in, 1 out]
                    n268 = vi-ref "断电保存全局.vi"() -> (w408:refnum<vi>)
                    n269 = call <userlib>:"Write Panel to INI__ogtk.vi"("error in (no error)"=w410, "VI ref"=w408, "refnum"=w407) -> ("error out"=w411:errorcluster, "refnum out"=w409:T10)  [unwired: 7 in]
                    n270 = call <vilib>:"Close Config Data.vi"("error in (no error)"=w411, "refnum"=w409) -> ("error out"=w416:errorcluster, "file path"=w417:path)  [unwired: 8 in]
                    n271 = Open/Create/Replace File(file path (use dialog)=w417, error in=w416) -> (refnum out=w413:refnum<file>, error out=w412:errorcluster)  [unwired: 4 in, 1 out]
                    n272 = Flush File(refnum=w413, error in=w412) -> (refnum out=w414:refnum<file>, error out=w415:errorcluster)
                    n273 = Close File(refnum=w414, error in=w415) -> ()  [unwired: 2 out]
                  }
                }
              }
            }
          }
          frame "数据组合发送" {
            n274 = Variant To Data(type=FALSE, Variant=w418) -> (data=w419:bool)  [unwired: 1 in, 1 out]
            n275 = global write "断电保存全局.vi" "数据组合发送"(w419) -> ()
            n276 = Two Button Dialog(message="勾选数据组合发送功能表示所有参数打包整点同时上传、则只能整点发送延时较高，\n不勾选则表示单参数分别上传、则实时性较好，确定更改数据组合发送功能吗？" ("消息")) -> (T button?=w422:bool)  [unwired: 2 in]
            n277 = case shown="假" w422 {
              tunnel: w421 -> [w425 _]
              frame False {
                n278 = Variant To Data(type=FALSE, Variant=w425) -> (data=w424:bool)  [unwired: 1 in, 1 out]
                n279 = global write "断电保存全局.vi" "数据组合发送"(w424) -> ()
              }
              frame True {
                n280 = flat-sequence {
                  frame #0 {
                  }
                  frame #1 {
                    n281 = call <vilib>:"Application Directory.vi"() -> ("Application Directory"=w427:path)
                    n282 = Build Path(base path=w427, name or relative path="data\\sys.ini" ("名称或相对路径")) -> (appended path=w429:path)
                    n283 = call <vilib>:"Open Config Data.vi"("configuration file path"=w429) -> ("error out"=w433:errorcluster, "refnum"=w430:T10)  [unwired: 8 in, 1 out]
                    n284 = vi-ref "断电保存全局.vi"() -> (w431:refnum<vi>)
                    n285 = call <userlib>:"Write Panel to INI__ogtk.vi"("error in (no error)"=w433, "VI ref"=w431, "refnum"=w430) -> ("error out"=w434:errorcluster, "refnum out"=w432:T10)  [unwired: 7 in]
                    n286 = call <vilib>:"Close Config Data.vi"("error in (no error)"=w434, "refnum"=w432) -> ("error out"=w439:errorcluster, "file path"=w440:path)  [unwired: 8 in]
                    n287 = Open/Create/Replace File(file path (use dialog)=w440, error in=w439) -> (refnum out=w436:refnum<file>, error out=w435:errorcluster)  [unwired: 4 in, 1 out]
                    n288 = Flush File(refnum=w436, error in=w435) -> (refnum out=w437:refnum<file>, error out=w438:errorcluster)
                    n289 = Close File(refnum=w437, error in=w438) -> ()  [unwired: 2 out]
                  }
                }
              }
            }
          }
          frame "2011发送" {
            n290 = Variant To Data(type=FALSE, Variant=w441) -> (data=w442:bool)  [unwired: 1 in, 1 out]
            n291 = global write "断电保存全局.vi" "2011发送"(w442) -> ()
            n292 = Two Button Dialog(message="2011表示实时数据上传，一般情况需要勾选，确定更改2011实时数据发送功能吗？" ("消息")) -> (T button?=w445:bool)  [unwired: 2 in]
            n293 = case shown="真" w445 {
              tunnel: w444 -> [w448 _]
              frame False {
                n294 = Variant To Data(type=FALSE, Variant=w448) -> (data=w447:bool)  [unwired: 1 in, 1 out]
                n295 = global write "断电保存全局.vi" "2011发送"(w447) -> ()
              }
              frame True {
                n296 = flat-sequence {
                  frame #0 {
                  }
                  frame #1 {
                    n297 = call <vilib>:"Application Directory.vi"() -> ("Application Directory"=w450:path)
                    n298 = Build Path(base path=w450, name or relative path="data\\sys.ini" ("名称或相对路径")) -> (appended path=w452:path)
                    n299 = call <vilib>:"Open Config Data.vi"("configuration file path"=w452) -> ("error out"=w456:errorcluster, "refnum"=w453:T10)  [unwired: 8 in, 1 out]
                    n300 = vi-ref "断电保存全局.vi"() -> (w454:refnum<vi>)
                    n301 = call <userlib>:"Write Panel to INI__ogtk.vi"("error in (no error)"=w456, "VI ref"=w454, "refnum"=w453) -> ("error out"=w457:errorcluster, "refnum out"=w455:T10)  [unwired: 7 in]
                    n302 = call <vilib>:"Close Config Data.vi"("error in (no error)"=w457, "refnum"=w455) -> ("error out"=w462:errorcluster, "file path"=w463:path)  [unwired: 8 in]
                    n303 = Open/Create/Replace File(file path (use dialog)=w463, error in=w462) -> (refnum out=w459:refnum<file>, error out=w458:errorcluster)  [unwired: 4 in, 1 out]
                    n304 = Flush File(refnum=w459, error in=w458) -> (refnum out=w460:refnum<file>, error out=w461:errorcluster)
                    n305 = Close File(refnum=w460, error in=w461) -> ()  [unwired: 2 out]
                  }
                }
              }
            }
          }
          frame "日志、参数发送" {
            n306 = Variant To Data(type=FALSE, Variant=w464) -> (data=w465:bool)  [unwired: 1 in, 1 out]
            n307 = global write "断电保存全局.vi" "日志、参数发送"(w465) -> ()
            n308 = Two Button Dialog(message="选择是否需要仪器日志、状态和告警信息上传，一般情况需要勾选，确定更改日志、参数发送功能吗？" ("消息")) -> (T button?=w468:bool)  [unwired: 2 in]
            n309 = case shown="真" w468 {
              tunnel: w467 -> [w471 _]
              frame False {
                n310 = Variant To Data(type=FALSE, Variant=w471) -> (data=w470:bool)  [unwired: 1 in, 1 out]
                n311 = global write "断电保存全局.vi" "日志、参数发送"(w470) -> ()
              }
              frame True {
                n312 = flat-sequence {
                  frame #0 {
                  }
                  frame #1 {
                    n313 = call <vilib>:"Application Directory.vi"() -> ("Application Directory"=w473:path)
                    n314 = Build Path(base path=w473, name or relative path="data\\sys.ini" ("名称或相对路径")) -> (appended path=w475:path)
                    n315 = call <vilib>:"Open Config Data.vi"("configuration file path"=w475) -> ("error out"=w479:errorcluster, "refnum"=w476:T10)  [unwired: 8 in, 1 out]
                    n316 = vi-ref "断电保存全局.vi"() -> (w477:refnum<vi>)
                    n317 = call <userlib>:"Write Panel to INI__ogtk.vi"("error in (no error)"=w479, "VI ref"=w477, "refnum"=w476) -> ("error out"=w480:errorcluster, "refnum out"=w478:T10)  [unwired: 7 in]
                    n318 = call <vilib>:"Close Config Data.vi"("error in (no error)"=w480, "refnum"=w478) -> ("error out"=w485:errorcluster, "file path"=w486:path)  [unwired: 8 in]
                    n319 = Open/Create/Replace File(file path (use dialog)=w486, error in=w485) -> (refnum out=w482:refnum<file>, error out=w481:errorcluster)  [unwired: 4 in, 1 out]
                    n320 = Flush File(refnum=w482, error in=w481) -> (refnum out=w483:refnum<file>, error out=w484:errorcluster)
                    n321 = Close File(refnum=w483, error in=w484) -> ()  [unwired: 2 out]
                  }
                }
              }
            }
          }
          frame "判断数据反馈" {
            n322 = Variant To Data(type=FALSE, Variant=w487) -> (data=w488:bool)  [unwired: 1 in, 1 out]
            n323 = global write "断电保存全局.vi" "判断数据反馈"(w488) -> ()
            n324 = Two Button Dialog(message="勾选判断数据反馈是针对平台能有反馈的情况、此功能能保证数据的完整性，尽可能的防止各种问题导致的数据缺失，\n不勾选则表示数据只发送不判断平台的反馈、用于针对平台没有反馈的情况，确定更改判断数据反馈功能吗？" ("消息")) -> (T button?=w491:bool)  [unwired: 2 in]
            n325 = case shown="真" w491 {
              tunnel: w490 -> [w494 _]
              frame False {
                n326 = Variant To Data(type=FALSE, Variant=w494) -> (data=w493:bool)  [unwired: 1 in, 1 out]
                n327 = global write "断电保存全局.vi" "判断数据反馈"(w493) -> ()
              }
              frame True {
                n328 = flat-sequence {
                  frame #0 {
                  }
                  frame #1 {
                    n329 = call <vilib>:"Application Directory.vi"() -> ("Application Directory"=w496:path)
                    n330 = Build Path(base path=w496, name or relative path="data\\sys.ini" ("名称或相对路径")) -> (appended path=w498:path)
                    n331 = call <vilib>:"Open Config Data.vi"("configuration file path"=w498) -> ("error out"=w502:errorcluster, "refnum"=w499:T10)  [unwired: 8 in, 1 out]
                    n332 = vi-ref "断电保存全局.vi"() -> (w500:refnum<vi>)
                    n333 = call <userlib>:"Write Panel to INI__ogtk.vi"("error in (no error)"=w502, "VI ref"=w500, "refnum"=w499) -> ("error out"=w503:errorcluster, "refnum out"=w501:T10)  [unwired: 7 in]
                    n334 = call <vilib>:"Close Config Data.vi"("error in (no error)"=w503, "refnum"=w501) -> ("error out"=w508:errorcluster, "file path"=w509:path)  [unwired: 8 in]
                    n335 = Open/Create/Replace File(file path (use dialog)=w509, error in=w508) -> (refnum out=w505:refnum<file>, error out=w504:errorcluster)  [unwired: 4 in, 1 out]
                    n336 = Flush File(refnum=w505, error in=w504) -> (refnum out=w506:refnum<file>, error out=w507:errorcluster)
                    n337 = Close File(refnum=w506, error in=w507) -> ()  [unwired: 2 out]
                  }
                }
              }
            }
          }
        }
      }
      event "确定": Value Change {
        n338 = event-data() -> ()  [unwired: 1 in, 6 out]
        n339 = call "通信状态入队列.vi"("枚举"=enum16{"打开连接", "发送数据", "读取数据", "数据处理", "关闭连接"}."关闭连接") -> ()  [unwired: 10 in, 1 out]
      }
      event "参数配置": Value Change {
        n340 = event-data() -> ()  [unwired: 1 in, 6 out]
        n341 = property on="窗格" class="Pane"("Origin"=T8 {"Horizontal"=0, "Vertical"=1000} ("原点")) -> ()  [unwired: 2 in, 2 out]
        n342 = call <vilib>:"Application Directory.vi"() -> ("Application Directory"=w512:path)
        n343 = call "查询启动项.vi"("启动文件路径"=w512) -> ("包含启动项"=w511:bool)  [unwired: 9 in, 1 out]
        n344 = local write "开机启动"(w511) -> ()
      }
      event "返回": Value Change {
        n345 = event-data() -> ()  [unwired: 1 in, 6 out]
        n346 = property on="窗格" class="Pane"("Origin"=T8 {"Horizontal"=0, "Vertical"=0} ("原点")) -> ()  [unwired: 2 in, 2 out]
      }
      event "确定更改起始时间": Value Change {
        n347 = event-data() -> ()  [unwired: 1 in, 6 out]
        n348 = local write "更改起始时间"(FALSE ("更改起始时间")) -> ()
        n349 = Two Button Dialog(message="确定以当前设置时间作为数据索引起始时间？" ("消息")) -> (T button?=w515:bool)  [unwired: 2 in]
        n350 = case shown="真" w515 {
          frame False {
          }
          frame True {
            n351 = global write "断电保存全局.vi" "数据重发"(TRUE ("数据重发")) -> ()
            n352 = Format Date/Time String(time format string (%c)="%Y/%m/%d %H:%M:%S" ("时间格式字符串(%c)"), seconds (now)="数据发送起始时间") -> (date/time string=w519:string)  [unwired: 1 in]
            n353 = global write "断电保存全局.vi" "数据重发时间戳"(w519) -> ()
            n354 = Initialize Array(w519, 27 ("维数大小")) -> (w520:string[])
            n355 = Array To Cluster(array=w520) -> (cluster=w518:T12)
            n356 = global write "全局 水样时间.vi" "水样数据索引"(w518) -> ()
            n357 = global read "断电保存全局.vi" "数据组合发送"() -> (w524:bool)
            n358 = case shown="假" w524 {
              tunnel: w519 -> [w526 _]
              frame False {
                n359 = global write "全局 时间2.vi" "标样核查索引起始时间"(w526) -> ()
                n360 = global write "全局 时间2.vi" "加标回收索引起始时间"(w526) -> ()
                n361 = global write "全局 时间2.vi" "跨度核查索引起始时间"(w526) -> ()
                n362 = global write "全局 时间2.vi" "零点核查索引起始时间"(w526) -> ()
                n363 = Initialize Array(w526, 8 ("维数大小")) -> (w532:string[])
                n364 = Initialize Array(w526, 15 ("维数大小")) -> (w527:string[])
                n365 = Array To Cluster(array=w532) -> (cluster=w531:T14)
                n366 = Array To Cluster(array=w527) -> (cluster=w528:T15)
                n367 = global write "全局 时间2.vi" "零点核查索引"(w531) -> ()
                n368 = global write "全局 时间2.vi" "跨度核查索引"(w531) -> ()
                n369 = global write "全局 时间2.vi" "标样核查索引"(w528) -> ()
                n370 = global write "全局 时间2.vi" "集成干预索引"(w528) -> ()
              }
              frame True {
              }
            }
          }
        }
      }
      event "开机启动": Value Change {
        n371 = event-data() -> ("CtlRef"=w534:refnum<vi>, "OldVal"=w533:bool, "NewVal"=w535:bool)  [unwired: 1 in, 3 out]
        n372 = case shown="真" w535 {
          tunnel: w534 -> [w537 w550]
          tunnel: w533 -> [w536 w549]
          frame False {
            n373 = Two Button Dialog(message="是否删除开机启动？" ("消息"), 1:"否" ("F按钮名称（“取消”）"), 2:"是" ("T按钮名称（“确定”）")) -> (T button?=w538:bool)
            n374 = case shown="假" w538 {
              tunnel: w537 -> [w543 _]
              tunnel: w536 -> [w542 _]
              frame False {
                n375 = property class="Bool (严格)"(reference=w543, "Value"=w542) -> ()  [unwired: 1 in, 2 out]
              }
              frame True {
                n376 = call <vilib>:"Application Directory.vi"() -> ("Application Directory"=w545:path)
                n377 = call "删除启动项.vi"("启动文件路径"=w545) -> ("删除标记"=w544:bool)  [unwired: 9 in, 1 out]
                n378 = case shown="假" w544 {
                  tunnel: ["删除开机启动失败" ("T按钮名称（“确定”）") "删除开机启动成功" ("T按钮名称（“确定”）")] -> w546
                  frame False {
                  }
                  frame True {
                  }
                }
                n379 = One Button Dialog(message=w546) -> ()  [unwired: 1 in, 1 out]
              }
            }
          }
          frame True {
            n380 = Two Button Dialog(message="是否添加开机启动？" ("消息"), 1:"否" ("F按钮名称（“取消”）"), 2:"是" ("T按钮名称（“确定”）")) -> (T button?=w551:bool)
            n381 = case shown="真" w551 {
              tunnel: w550 -> [w556 _]
              tunnel: w549 -> [w555 _]
              frame False {
                n382 = property class="Bool (严格)"(reference=w556, "Value"=w555) -> ()  [unwired: 1 in, 2 out]
              }
              frame True {
                n383 = call <vilib>:"Application Directory.vi"() -> ("Application Directory"=w559:path)
                n384 = call "添加启动项.vi"("启动文件路径"=w559) -> ("添加成功标记"=w558:bool)  [unwired: 9 in, 1 out]
                n385 = case shown="真" w558 {
                  tunnel: ["添加开机启动失败" ("T按钮名称（“确定”）") "添加开机启动成功" ("T按钮名称（“确定”）")] -> w557
                  frame False {
                  }
                  frame True {
                  }
                }
                n386 = One Button Dialog(message=w557) -> ()  [unwired: 1 in, 1 out]
              }
            }
          }
        }
      }
      event "更新": Value Change {
        n387 = event-data() -> ()  [unwired: 1 in, 6 out]
        n388 = call "自定义双按钮对话框.vi"("消息"="选择是否从服务器获取最新版本信息？") -> ("输出"=w562:bool)  [unwired: 10 in]
        n389 = case shown="真" w562 {
          frame False {
          }
          frame True {
            # "获取最新版本"
            n390 = disable-structure shown="禁用" {
              frame Disabled {
                n391 = call "FTP自动升级更新main.vi"() -> ()  [unwired: 12 in]
              }
              frame Enabled {
              }
            }
          }
        }
      }
      event "updateconfiguration": Value Change {
        n392 = event-data() -> ("NewVal"=w571:T1)  [unwired: 1 in, 5 out]
        n393 = call <vilib>:"Application Directory.vi"() -> ("Application Directory"=w575:path)
        n394 = Build Array("主机" ("section"), "用户" ("section"), "密码" ("key"), "远程路径" ("key"), "下载文件名" ("key"), "软件版本" ("key")) -> (w564:string[])
        n395 = Build Path(base path=w575, name or relative path="update\\data\\set.ini" ("名称或相对路径")) -> (appended path=w573:path)
        n396 = call "配置文件write.vi"("updateconfiguration"=w571, "configuration file path"=w573, "键数组"=w564, "段"="应用程序交互" ("section")) -> ("error out"=w572:errorcluster)  [unwired: 7 in]
        n397 = call <vilib>:"Clear Errors.vi"("error in (no error)"=w572) -> ()  [unwired: 5 in, 2 out]
      }
      event "IP", "PORT": Mouse Down {
        n398 = event-data() -> ("CtlRef"=w580:refnum<vi>)  [unwired: 1 in, 7 out]
        n399 = property class="Str"(reference=w580) -> (reference out=w578:refnum<vi>, "Value"=w579:string)  [unwired: 1 in, 1 out]
        n400 = call "IP键盘.vi"("OldNumber"=w579) -> ("NewNumber"=w577:string)
        n401 = property class="Str"(reference=w578, "Val(Sgnl)"=w577) -> ()  [unwired: 1 in, 2 out]
      }
    }
  }
  n402 = disable-structure shown="启用" {
    disable-tunnel: [w582 T16."Standard" ("状态")] -> w69
    disable-tunnel: w46 -> [w581 _]
    frame Disabled {
      n403 = case shown="\"Development System\", 默认" w581 {
        tunnel: [T16."Standard" ("状态") T16."Hidden" ("状态")] -> w582
        frame "Development System", Default {
        }
        frame "Run Time System" {
        }
      }
    }
    frame Enabled {
    }
  }
  n404 = Obtain Queue(name (unnamed)="actualwrite" ("名称（未命名）"), element data type=enum16{"打开连接", "发送数据", "读取数据", "数据处理", "关闭连接"}."打开连接" ("枚举")) -> (queue out=w25:refnum<queue>, error out=w24:errorcluster)  [unwired: 3 in, 1 out]
  n405 = Obtain Queue(name (unnamed)="actualread" ("名称（未命名）"), element data type=enum16{"打开连接", "发送数据", "读取数据", "数据处理", "关闭连接"}."打开连接" ("枚举")) -> (queue out=w22:refnum<queue>, error out=w15:errorcluster)  [unwired: 3 in, 1 out]
  n406 = property class="VI"(reference=w37) -> ("Name"=w36:string)  [unwired: 1 in, 2 out]
  n407 = property class="VI"(reference=w38) -> ("Name"=w45:string)  [unwired: 1 in, 2 out]
  n408 = while {
    tunnel: w25 -> [w594]
    tunnel: w24 -> [w593]
    shift-right: [w589] -> _
    shift-left: errorcluster {"status"=FALSE, "code"=0, "source"=""} ("error out") -> [w588]
    stop <- FALSE stop-if-true
    # "写入数据出队列"
    n409 = Dequeue Element(queue=w594, timeout in ms (-1)=30000 ("超时毫秒(-1)"), error in (no error)=w593) -> (queue out=w587:refnum<queue>, element=w591:enum16{"打开连接", "发送数据", "读取数据", "数据处理", "关闭连接"}, timed out?=w590:bool, error out=w586:errorcluster)
    n410 = case shown="无错误" w588 {
      tunnel: w591 -> [w596 _]
      tunnel: w590 -> [w598 _]
      tunnel: [w602 w643] -> w589
      tunnel: w588 -> [w601 w647]
      tunnel: w587 -> [w600 w645]
      tunnel: w586 -> [w599 w644]
      frame No Error {
        n411 = case shown="假" w598 {
          tunnel: [w603 enum16{"打开连接", "发送数据", "读取数据", "数据处理", "关闭连接"}."发送数据" ("枚举")] -> w597
          tunnel: w596 -> [w603 _]
          frame False {
          }
          frame True {
          }
        }
        n412 = case shown="\"发送数据\", 默认" w597 {
          tunnel: w598 -> [_ w620 _ _ _]
          tunnel: [w606 w615 _ _ w636] -> w602
          tunnel: w601 -> [w608 w622 _ _ w637]
          tunnel: w600 -> [_ _ _ _ w638]
          tunnel: w599 -> [_ _ _ _ w635]
          frame "打开连接" {
            n413 = global read "断电保存全局.vi" "VISA resource name"() -> (w614:refnum<visa-resource-name>)
            n414 = global read "断电保存全局.vi" "数据发送通道"() -> (w611:enum16{"TCP", "VISA"})
            n415 = global read "断电保存全局.vi" "baud rate"() -> (w613:u32)
            n416 = global read "断电保存全局.vi" "PORT"() -> (w612:string)
            n417 = global read "断电保存全局.vi" "IP"() -> (w610:string)
            n418 = call "VISATCP组合选择发送.vi"("IP"=w610, "数据发送通道"=w611, "命令"="open", "PORT"=w612, "VISA resource name"=w614, "baud rate"=w613, "error in (no error)"=w608) -> ("错误输出"=w606:errorcluster)  [unwired: 5 in, 3 out]
            n419 = Unbundle By Name(w606) -> ("status"=w605:bool)  [unwired: 1 out]
            n420 = Not(x=w605) -> (.not. x?=w607:bool)
            n421 = global write "全局 数据发送重叠.vi" "掉线指示灯"(w605) -> ()
            n422 = local write "通信状态"(w607) -> ()
          }
          frame "发送数据", Default {
            n423 = case shown="真" w620 {
              tunnel: [w627 w629] -> w617
              tunnel: w622 -> [w626 w630]
              tunnel: [w626 w630] -> w621
              frame False {
                # "事件触发发送数据"
                n424 = global read "全局1.vi" "发送报文显示"() -> (w627:string)
              }
              frame True {
                # "30秒超时发送心跳包"
                n425 = local read "配置信息"() -> (w633:T5)
                n426 = Unbundle By Name(w633) -> ("MN"=w632:string, "PW"=w631:string)
                n427 = call "数据编码.vi"("table输入"="心跳包", "MN"=w632, "PW"=w631) -> ("通讯包字符串"=w629:string)  [unwired: 11 in, 1 out]
                n428 = global write "全局1.vi" "发送报文显示"(w629) -> ()
                n429 = Wait (ms)(milliseconds to wait=u32 500 ("等待时间（毫秒）")) -> ()  [unwired: 1 out]
              }
            }
            n430 = global read "断电保存全局.vi" "数据发送通道"() -> (w623:enum16{"TCP", "VISA"})
            n431 = Concatenate Strings("send:" ("字符串"), w617) -> (w616:string)
            n432 = call "VISATCP组合选择发送.vi"("数据发送通道"=w623, "命令"="write", "error in (no error)"=w621, "写入缓冲区"=w617) -> ("错误输出"=w615:errorcluster)  [unwired: 8 in, 3 out]
            n433 = Build Array(w616) -> (w619:string[])
            n434 = call "发送数据记录到文档(子VI).vi"("数组"=w619) -> ()  [unwired: 9 in, 1 out]
            n435 = flat-sequence {
              tunnel: w615 -> [_]
              frame #0 {
                n436 = local write "心跳包"(FALSE ("心跳包")) -> ()
              }
            }
            "心跳包" <- w620
          }
          frame "读取数据" {
          }
          frame "数据处理" {
          }
          frame "关闭连接" {
            n437 = global read "断电保存全局.vi" "数据发送通道"() -> (w640:enum16{"TCP", "VISA"})
            n438 = Enqueue Element(queue=w638, element=enum16{"打开连接", "发送数据", "读取数据", "数据处理", "关闭连接"}."打开连接" ("枚举"), error in (no error)=w635) -> ()  [unwired: 1 in, 3 out]
            n439 = call "VISATCP组合选择发送.vi"("数据发送通道"=w640, "命令"="close", "error in (no error)"=w637) -> ("错误输出"=w641:errorcluster)  [unwired: 9 in, 3 out]
            n440 = call <vilib>:"Clear Errors.vi"("error in (no error)"=w641) -> ("error out"=w636:errorcluster)  [unwired: 5 in, 1 out]
          }
        }
      }
      frame Error {
        n441 = Unbundle By Name(w647) -> ("code"=w646:i32)
        n442 = case shown="0, 默认" w646 {
          tunnel: w645 -> [w654 w670 w682]
          tunnel: w644 -> [w653 w669 w681]
          tunnel: [w652 w667 w680] -> w643
          frame 0, Default {
            n443 = Flush Queue(queue=w654, error in (no error)=w653) -> (queue out=w656:refnum<queue>, error out=w657:errorcluster)  [unwired: 1 out]
            n444 = local read "状态信息"() -> (w651:T4)
            n445 = Unbundle By Name(w651) -> ("TCP服务端掉线计数"=w649:i32)
            n446 = Enqueue Element(queue=w656, element=enum16{"打开连接", "发送数据", "读取数据", "数据处理", "关闭连接"}."关闭连接" ("枚举"), error in (no error)=w657) -> (error out=w658:errorcluster)  [unwired: 1 in, 2 out]
            n447 = Increment(x=w649) -> (x+1=w650:i32)
            n448 = Bundle By Name(cluster=w651, "TCP服务端掉线计数"=w650) -> (w648:T4)
            n449 = local write "状态信息"(w648) -> ()
            n450 = call <vilib>:"Clear Errors.vi"("error in (no error)"=w658) -> ("error out"=w652:errorcluster)  [unwired: 5 in, 1 out]
          }
          frame 54, 63 {
            n451 = Flush Queue(queue=w670, error in (no error)=w669) -> (queue out=w672:refnum<queue>, error out=w673:errorcluster)  [unwired: 1 out]
            n452 = local read "状态信息"() -> (w662:T4)
            n453 = Unbundle By Name(w662) -> ("TCP服务端掉线计数"=w666:i32, "TCP掉线时间节点"=w659:string)
            n454 = Enqueue Element(queue=w672, element=enum16{"打开连接", "发送数据", "读取数据", "数据处理", "关闭连接"}."关闭连接" ("枚举"), error in (no error)=w673) -> (error out=w668:errorcluster)  [unwired: 1 in, 2 out]
            n455 = Less Or Equal?(x=w666, y=1) -> (x <= y?=w664:bool)
            n456 = case shown="真" w664 {
              tunnel: [w674 w675] -> w663
              tunnel: w659 -> [w674 _]
              frame False {
              }
              frame True {
                n457 = Get Date/Time In Seconds() -> (seconds since 1Jan1904=w676:timestamp)
                n458 = Format Date/Time String(time format string (%c)="%Y%m%d%H%M%S%3u" ("时间格式字符串(%c)"), seconds (now)=w676) -> (date/time string=w678:string)  [unwired: 1 in]
                n459 = call "格式时间字符串.vi"("字符串"=w678) -> ("连接的字符串"=w675:string)  [unwired: 10 in]
              }
            }
            n460 = Increment(x=w666) -> (x+1=w661:i32)
            n461 = call <vilib>:"Clear Errors.vi"("error in (no error)"=w668) -> ("error out"=w667:errorcluster)  [unwired: 5 in, 1 out]
            n462 = Bundle By Name(cluster=w662, "TCP服务端掉线计数"=w661, "TCP掉线时间节点"=w663) -> (w660:T4)
            n463 = local write "状态信息"(w660) -> ()
          }
          frame 56 {
            n464 = Flush Queue(queue=w682, error in (no error)=w681) -> (error out=w679:errorcluster)  [unwired: 2 out]
            n465 = call <vilib>:"Clear Errors.vi"("error in (no error)"=w679) -> ("error out"=w680:errorcluster)  [unwired: 5 in, 1 out]
          }
        }
      }
    }
  }
  n466 = call <vilib>:"Application Directory.vi"() -> ("Application Directory"=w52:path)
  n467 = property class="App"() -> ("App.Name"=w4:string)  [unwired: 2 in, 2 out]
  n468 = Open VI Reference(type specifier VI Refnum (for type only)=refnum<vi> refnum, vi path=w36, options=128 ("选项")) -> (vi reference=w34:refnum<vi>, error out=w32:errorcluster)  [unwired: 3 in]
  n469 = Open VI Reference(type specifier VI Refnum (for type only)=refnum<vi> refnum, vi path=w45, options=128 ("选项")) -> (vi reference=w43:refnum<vi>, error out=w41:errorcluster)  [unwired: 3 in]
  n470 = Obtain Queue(name (unnamed)="反控命令信息队列" ("名称（未命名）"), element data type=cluster{"命令编码CN":string, "QN":string} {"命令编码CN"="", "QN"=""}) -> (queue out=w9:refnum<queue>, error out=w8:errorcluster)  [unwired: 3 in, 1 out]
  n471 = Build Path(base path=w52, name or relative path="data\\tubiao.ico" ("名称或相对路径")) -> (appended path=w60:path)
  n472 = Enqueue Element(queue=w22, element=enum16{"打开连接", "发送数据", "读取数据", "数据处理", "关闭连接"}."打开连接" ("枚举"), error in (no error)=w15) -> (queue out=w18:refnum<queue>, error out=w17:errorcluster)  [unwired: 1 in, 1 out]
  n473 = Obtain Queue(name (unnamed)="datasent" ("名称（未命名）"), element data type="实时小时数据" ("元素")) -> (queue out=w13:refnum<queue>, error out=w12:errorcluster)  [unwired: 3 in, 1 out]
  n474 = Current VI's Path() -> (path=w49:path)
  n475 = call-by-ref "?"(reference=w34, error in=w32) -> (reference out=w30:refnum<vi>, error out=w31:errorcluster)  [unwired: 12 in]
  n476 = call-by-ref "?"(reference=w43, error in=w41) -> (reference out=w39:refnum<vi>, error out=w40:errorcluster)  [unwired: 12 in]
  n477 = Build Array(w60) -> (w55:path[])
  n478 = Open VI Reference(vi path=w49) -> (vi reference=w48:refnum<vi>)  [unwired: 5 in, 1 out]
  n479 = Close Reference(reference=w30, error in (no error)=w31) -> ()  [unwired: 1 out]
  n480 = Close Reference(reference=w39, error in (no error)=w40) -> ()  [unwired: 1 out]
  n481 = invoke class="VI" method="FP.Open"(reference=w48, "Activate"=TRUE ("激活？"), "State"=w69) -> (error out=w47:errorcluster)  [unwired: 2 in, 4 out]
  n482 = while {
    tunnel: w18 -> [w695]
    tunnel: w17 -> [w694]
    shift-right: [w691] -> _
    shift-left: errorcluster {"status"=FALSE, "code"=0, "source"=""} ("error out") -> [w690]
    tunnel: w13 -> [w686]
    tunnel: w12 -> [w685]
    tunnel: w9 -> [w684]
    tunnel: w8 -> [w683]
    stop <- FALSE stop-if-true
    # "读取数据出队列处理"
    n483 = Dequeue Element(queue=w695, error in (no error)=w694) -> (queue out=w689:refnum<queue>, element=w692:enum16{"打开连接", "发送数据", "读取数据", "数据处理", "关闭连接"}, error out=w688:errorcluster)  [unwired: 1 in, 1 out]
    n484 = Wait (ms)(milliseconds to wait=u32 1000 ("等待时间（毫秒）")) -> ()  [unwired: 1 out]
    n485 = case shown="无错误" w690 {
      tunnel: w692 -> [w701 _]
      tunnel: [w708 w786] -> w691
      tunnel: w690 -> [w707 w790]
      tunnel: w689 -> [w706 w788]
      tunnel: w688 -> [w705 w787]
      tunnel: w686 -> [w699 _]
      tunnel: w685 -> [w698 _]
      tunnel: w684 -> [w697 _]
      tunnel: w683 -> [w696 _]
      frame No Error {
        n486 = case shown="\"打开连接\", 默认" w701 {
          tunnel: [w715 _ w749 _ w781] -> w708
          tunnel: w707 -> [w714 _ w752 _ w782]
          tunnel: w706 -> [w712 _ w744 _ w779]
          tunnel: w705 -> [w711 _ w743 _ w778]
          tunnel: [w710 _ _ _ _] -> w702
          tunnel: w699 -> [_ _ w736 _ _]
          tunnel: w698 -> [_ _ w735 _ _]
          tunnel: w697 -> [_ _ w724 _ _]
          tunnel: w696 -> [_ _ w723 _ _]
          frame "打开连接", Default {
            n487 = Enqueue Element(queue=w712, element=enum16{"打开连接", "发送数据", "读取数据", "数据处理", "关闭连接"}."读取数据" ("枚举"), error in (no error)=w711) -> ()  [unwired: 1 in, 3 out]
            n488 = global read "断电保存全局.vi" "VISA resource name"() -> (w722:refnum<visa-resource-name>)
            n489 = global read "断电保存全局.vi" "数据发送通道"() -> (w719:enum16{"TCP", "VISA"})
            n490 = global read "断电保存全局.vi" "baud rate"() -> (w721:u32)
            n491 = global read "断电保存全局.vi" "PORT"() -> (w720:string)
            n492 = global read "断电保存全局.vi" "IP"() -> (w718:string)
            n493 = call "VISATCP组合选择发送.vi"("IP"=w718, "数据发送通道"=w719, "命令"="open", "PORT"=w720, "VISA resource name"=w722, "baud rate"=w721, "error in (no error)"=w714) -> ("错误输出"=w715:errorcluster)  [unwired: 5 in, 3 out]
            n494 = Unbundle By Name(w715) -> ("status"=w709:bool, "code"=w710:i32)
            n495 = Not(x=w709) -> (.not. x?=→"通信状态":bool)
            n496 = global write "全局 数据发送重叠.vi" "掉线指示灯"(w709) -> ()
          }
          frame "发送数据" {
          }
          frame "读取数据" {
            n497 = Get Queue Status(queue=w744, error in (no error)=w743) -> (queue out=w740:refnum<queue>, error out=w739:errorcluster, # elements in queue=w742:i32)  [unwired: 1 in, 5 out]
            n498 = global read "断电保存全局.vi" "数据发送通道"() -> (w751:enum16{"TCP", "VISA"})
            n499 = Equal To 0?(x=w742) -> (x = 0?=w741:bool)
            n500 = case shown="真" w741 {
              tunnel: w740 -> [_ w776]
              tunnel: w739 -> [_ w775]
              frame False {
              }
              frame True {
                n501 = Enqueue Element(queue=w776, element=enum16{"打开连接", "发送数据", "读取数据", "数据处理", "关闭连接"}."读取数据" ("枚举"), error in (no error)=w775) -> ()  [unwired: 1 in, 3 out]
              }
            }
            n502 = call "VISATCP组合选择发送.vi"("数据发送通道"=w751, "命令"="read", "error in (no error)"=w752) -> ("读取缓冲区"=w737:string, "错误输出"=w749:errorcluster)  [unwired: 9 in, 2 out]
            n503 = call "读取数据处理 (子VI).vi"("data out"=w737) -> ("命令编码CN"=w745:string, "数据"=w733:string, "时间QN"=w725:string)  [unwired: 8 in, 4 out]
            n504 = Empty String/Path?(string/path=w737) -> (empty?=w738:bool)
            n505 = case shown="假" w738 {
              tunnel: w737 -> [w772 _]
              tunnel: w725 -> [w769 _]
              frame False {
                n506 = Search/Split String(string=w769, search string/char (-)="QN=" ("搜索字符串/字符(-)")) -> (match + rest of string=w768:string)  [unwired: 1 in, 2 out]
                n507 = global write "全局1.vi" "数据输出"(w772) -> ()
                n508 = global write "全局1.vi" "读取报文显示"(w772) -> ()
                n509 = String Subset(string=w768, offset (0)=3 ("偏移量(0)")) -> (substring=w767:string)  [unwired: 1 in]
                n510 = global write "全局1.vi" "QN"(w767) -> ()
                n511 = call "数据记录.vi"("写入字段"=w772) -> ("连接的字符串"=w773:string)  [unwired: 10 in]
                n512 = Build Array(w773) -> (w774:string[])
                n513 = call "发送数据记录到文档(子VI).vi"("数组"=w774) -> ()  [unwired: 9 in, 1 out]
              }
              frame True {
              }
            }
            n514 = Search/Split String(string=w745, search string/char (-)="CN=" ("搜索字符串/字符(-)")) -> (match + rest of string=w746:string)  [unwired: 1 in, 2 out]
            n515 = String Subset(string=w746, offset (0)=3 ("偏移量(0)")) -> (substring=w731:string)  [unwired: 1 in]
            n516 = Empty String/Path?(string/path=w731) -> (empty?=w734:bool)
            n517 = Not Equal?(x=w731, y="9013") -> (x != y?=w728:bool)
            n518 = Not Equal?(x=w731, y="9014") -> (x != y?=w727:bool)
            n519 = Not(x=w734) -> (.not. x?=w726:bool)
            n520 = Compound Arithmetic op=AND ("复合运算")(w726, w728, w727) -> (w732:bool)
            n521 = case shown="真" w732 {
              tunnel: w736 -> [_ w766]
              tunnel: w735 -> [_ w765]
              tunnel: w733 -> [_ w764]
              tunnel: w731 -> [_ w755]
              tunnel: w725 -> [_ w760]
              tunnel: w724 -> [_ w759]
              tunnel: w723 -> [_ w758]
              frame False {
              }
              frame True {
                n522 = global write "全局1.vi" "数据"(w764) -> ()
                n523 = Search/Split String(string=w760, search string/char (-)="QN=" ("搜索字符串/字符(-)")) -> (match + rest of string=w763:string)  [unwired: 1 in, 2 out]
                n524 = global write "全局1.vi" "命令编码CN"(w755) -> ()
                n525 = String Subset(string=w763, offset (0)=3 ("偏移量(0)")) -> (substring=w754:string)  [unwired: 1 in]
                n526 = Bundle By Name(cluster=cluster{"命令编码CN":string, "QN":string} {"命令编码CN"="", "QN"=""}, "命令编码CN"=w755, "QN"=w754) -> (w756:cluster{"命令编码CN":string, "QN":string})
                n527 = Enqueue Element At Opposite End(queue=w766, element="反控命令" ("元素"), error in (no error)=w765) -> ()  [unwired: 1 in, 3 out]
                n528 = Enqueue Element(queue=w759, element=w756, error in (no error)=w758) -> ()  [unwired: 1 in, 3 out]
              }
            }
          }
          frame "数据处理" {
          }
          frame "关闭连接" {
            n529 = global read "断电保存全局.vi" "数据发送通道"() -> (w784:enum16{"TCP", "VISA"})
            n530 = Enqueue Element(queue=w779, element=enum16{"打开连接", "发送数据", "读取数据", "数据处理", "关闭连接"}."打开连接" ("枚举"), error in (no error)=w778) -> ()  [unwired: 1 in, 3 out]
            n531 = call "VISATCP组合选择发送.vi"("数据发送通道"=w784, "命令"="close", "error in (no error)"=w782) -> ("错误输出"=w783:errorcluster)  [unwired: 9 in, 3 out]
            n532 = call <vilib>:"Clear Errors.vi"("error in (no error)"=w783) -> ("error out"=w781:errorcluster)  [unwired: 5 in, 1 out]
          }
        }
        n533 = local read "状态信息"() -> (w704:T4)
        n534 = Bundle By Name(cluster=w704, "TCP服务端掉线计数"=0, "1st Error to Convert"=w702, "步骤"=w701) -> (→"状态信息":T4)
      }
      frame Error {
        n535 = Unbundle By Name(w790) -> ("code"=w789:i32)
        n536 = case shown="54, 63" w789 {
          tunnel: w788 -> [w797 w813 w824]
          tunnel: w787 -> [w796 w812 w823]
          tunnel: [w795 w810 w822] -> w786
          frame 0, Default {
            n537 = Flush Queue(queue=w797, error in (no error)=w796) -> (queue out=w799:refnum<queue>, error out=w800:errorcluster)  [unwired: 1 out]
            n538 = local read "状态信息"() -> (w794:T4)
            n539 = Enqueue Element(queue=w799, element=enum16{"打开连接", "发送数据", "读取数据", "数据处理", "关闭连接"}."关闭连接" ("枚举"), error in (no error)=w800) -> (error out=w801:errorcluster)  [unwired: 1 in, 2 out]
            n540 = Unbundle By Name(w794) -> ("TCP服务端掉线计数"=w792:i32)
            n541 = Increment(x=w792) -> (x+1=w793:i32)
            n542 = Bundle By Name(cluster=w794, "TCP服务端掉线计数"=w793) -> (w791:T4)
            n543 = local write "状态信息"(w791) -> ()
            n544 = call <vilib>:"Clear Errors.vi"("error in (no error)"=w801) -> ("error out"=w795:errorcluster)  [unwired: 5 in, 1 out]
          }
          frame 54, 63 {
            n545 = Flush Queue(queue=w813, error in (no error)=w812) -> (queue out=w815:refnum<queue>, error out=w816:errorcluster)  [unwired: 1 out]
            n546 = local read "状态信息"() -> (w805:T4)
            n547 = Unbundle By Name(w805) -> ("TCP服务端掉线计数"=w809:i32, "TCP掉线时间节点"=w802:string)
            n548 = Enqueue Element(queue=w815, element=enum16{"打开连接", "发送数据", "读取数据", "数据处理", "关闭连接"}."关闭连接" ("枚举"), error in (no error)=w816) -> (error out=w811:errorcluster)  [unwired: 1 in, 2 out]
            n549 = Less Or Equal?(x=w809, y=1) -> (x <= y?=w807:bool)
            n550 = Increment(x=w809) -> (x+1=w804:i32)
            n551 = case shown="真" w807 {
              tunnel: [w817 w818] -> w806
              tunnel: w802 -> [w817 _]
              frame False {
              }
              frame True {
                n552 = Get Date/Time In Seconds() -> (seconds since 1Jan1904=w819:timestamp)
                n553 = Format Date/Time String(time format string (%c)="%Y%m%d%H%M%S%3u" ("时间格式字符串(%c)"), seconds (now)=w819) -> (date/time string=w821:string)  [unwired: 1 in]
                n554 = call "格式时间字符串.vi"("字符串"=w821) -> ("连接的字符串"=w818:string)  [unwired: 10 in]
              }
            }
            n555 = call <vilib>:"Clear Errors.vi"("error in (no error)"=w811) -> ("error out"=w810:errorcluster)  [unwired: 5 in, 1 out]
            n556 = Bundle By Name(cluster=w805, "TCP服务端掉线计数"=w804, "TCP掉线时间节点"=w806) -> (w803:T4)
            n557 = local write "状态信息"(w803) -> ()
          }
          frame 56 {
            n558 = Flush Queue(queue=w824, error in (no error)=w823) -> (queue out=w826:refnum<queue>, error out=w827:errorcluster)  [unwired: 1 out]
            n559 = Enqueue Element(queue=w826, element=enum16{"打开连接", "发送数据", "读取数据", "数据处理", "关闭连接"}."读取数据" ("枚举"), error in (no error)=w827) -> (error out=w828:errorcluster)  [unwired: 1 in, 2 out]
            n560 = call <vilib>:"Clear Errors.vi"("error in (no error)"=w828) -> ("error out"=w822:errorcluster)  [unwired: 5 in, 1 out]
          }
        }
      }
    }
  }
  n561 = Build Array("Open", w4, "Exit" ("元素")) -> (w2:string[])
  n562 = call <vilib>:"Constructor.vi"("error in"=w47, "IconFilePathList"=w55) -> ("error out"=w59:errorcluster, "NotifyIcon"=w53:refnum<class "NotifyIcon.lvclass">)  [unwired: 8 in]
  n563 = for {
    shift-right: [w833] -> w71
    shift-left: w59 -> [w834]
    tunnel: w2 -> [w832] mode=indexing
    tunnel: w1 -> [w831] mode=indexing
    shift-right: [w829] -> w70
    shift-left: w53 -> [w830]
    # "2."
    n564 = call <vilib>:"InsertMenuItem.vi"("error in"=w834, "ItemTag"=w831, "ItemName"=w832, "NotifyIcon in"=w830) -> ("error out"=w833:errorcluster, "NotifyIcon out"=w829:refnum<class "NotifyIcon.lvclass">)  [unwired: 6 in]
  }
  n565 = Index Array(array=w1) -> (element=w54:string)  [unwired: 1 in]
  n566 = property class="NotifyIcon"(reference=w70, error in=w71, "Public:Visible"=TRUE ("Visible"), "Public:DefaultMenuItem"=w54, "Public:TipText"="平台数据传输系统" ("TipText")) -> (reference out=w67:refnum<class "NotifyIcon.lvclass">, error out=w58:errorcluster, "Public:SelectedItemEvent"=w57:refnum<user-event>)
  n567 = register-events(error in=w58, w57) -> (reference out=w28:refnum<event-registration>, error out=w29:errorcluster)  [unwired: 1 in]
  n568 = while {
    shift-right: [w838] -> w65
    shift-left: w29 -> [w837]
    shift-right: [w839] -> w62
    shift-left: w67 -> [w840]
    shift-right: [w836] -> w63
    shift-left: w28 -> [w841]
    tunnel: [w835] -> _
    stop <- w835 stop-if-true
    n569 = case shown="无错误" w837 {
      selector: w837 -> [w843 w878]
      tunnel: w841 -> [w848 w873]
      tunnel: w840 -> [w847 w874]
      tunnel: [w846 w874] -> w839
      tunnel: [w845 w876] -> w838
      tunnel: [w844 FALSE ("Discard?")] -> w835
      tunnel: [w842 w873] -> w836
      frame No Error {
        n570 = event shown="[0] <Public:SelectedItemEvent>: 用户事件" {
          selector: w848 -> [_ _ _]
          dyn-events: [_ _ _] -> w842
          timeout: _ -> [_ _ _]
          tunnel: w843 -> [w851 w862 w871]
          tunnel: [w851 w862 w870] -> w845
          tunnel: [w850 TRUE FALSE ("Discard?")] -> w844
          tunnel: w847 -> [w849 w860 w872]
          tunnel: [w849 w860 w869] -> w846
          event User Event {
            # "5."
            n571 = event-data() -> ("ItemTag"=w852:string)  [unwired: 1 in]
            n572 = case shown="默认" w852 {
              tunnel: [FALSE TRUE] -> w850
              frame Default {
                n573 = Current VI's Path() -> (path=w854:path)
                n574 = Open VI Reference(vi path=w854) -> (vi reference=w855:refnum<vi>)  [unwired: 5 in, 1 out]
                n575 = invoke class="VI" method="FP.Open"(reference=w855, "Activate"=TRUE ("激活？"), "State"=T16."Standard" ("状态")) -> ()  [unwired: 2 in, 5 out]
              }
              frame "EXIT" {
              }
            }
          }
          event "停止输入": Value Change {
            # "5."
            n576 = event-data() -> ()  [unwired: 1 in, 6 out]
            n577 = Stop(stop? (T)=TRUE ("可见")) -> ()
          }
          event Panel Close? {
            # "4."
            n578 = event-data() -> ("VIRef"=w865:refnum<vi>)  [unwired: 1 in, 3 out]
            n579 = invoke class="VI" method="FP.Open"(reference=w865, "State"=T16."Hidden" ("状态")) -> ()  [unwired: 3 in, 5 out]
            n580 = call <vilib>:"ShowBalloonTip.vi"("Balloon Icon"=BalloonIcon."Information", "error in"=w871, "Text"="欢迎使用平台数据传输系统", "NotifyIcon in"=w872) -> ("error out"=w870:errorcluster, "NotifyIcon out"=w869:refnum<class "NotifyIcon.lvclass">)  [unwired: 6 in]
            n581 = event-data("Discard?"=TRUE ("放弃？")) -> ()  [unwired: 1 in, 1 out]
          }
        }
      }
      frame Error {
        n582 = call <vilib>:"Simple Error Handler.vi"("error in (no error)"=w878) -> ("error out"=w877:errorcluster)  [unwired: 4 in, 4 out]
        n583 = call <vilib>:"Clear Errors.vi"("error in (no error)"=w877) -> ("error out"=w876:errorcluster)  [unwired: 5 in, 1 out]
      }
    }
  }
  n584 = Unregister For Events(event registration refnum=w63, error in=w65) -> (error out=w66:errorcluster)
  n585 = call <vilib>:"Destructor.vi"("error in"=w66, "NotifyIcon"=w62) -> ("error out"=w61:errorcluster)  [unwired: 9 in]
  n586 = call <vilib>:"Simple Error Handler.vi"("error in (no error)"=w61) -> ("error out"=→"错误输出":errorcluster)  [unwired: 4 in, 4 out]
  n587 = case shown="\"Run Time System\"" w46 {
    tunnel: w61 -> [_ _ _ _ _ _ _]
    frame "invalid app kind", Default {
    }
    frame "Development System" {
      n588 = Stop(stop? (T)=TRUE ("可见")) -> ()
    }
    frame "Run Time System" {
      n589 = Quit LabVIEW(quit? (T)=TRUE ("退出？(T)")) -> ()
    }
    frame "Student Edition" {
    }
    frame "Embedded LabVIEW" {
    }
    frame "Evaluation" {
    }
    frame "Custom" {
    }
  }
